vi "can test.vi"() -> ()   [LabVIEW 2015]
uses:
  <vilib>/myRIO/Instrument Drivers/Onboard IO/DIO/typedefs/DIO Reference.ctl
  <vilib>/myRIO/Common/Instrument Driver Framework/Utilities/typedefs/myRIO Generic Hardware Reference.ctl
  <vilib>/myRIO/Common/Instrument Driver Framework/Utilities/typedefs/Hardware Version Enum.ctl
  <vilib>/myRIO/Common/Instrument Driver Framework/Utilities/typedefs/myRIO v1.0 Reference.ctl
  <vilib>/myRIO/Common/Instrument Driver Framework/Utilities/typedefs/Generic FPGA Reference.ctl
  <vilib>/myRIO/Common/Instrument Driver Framework/myRIO v1.0/DIO/typedefs/DIO Channels List.ctl
  <vilib>/myRIO/Common/Instrument Driver Framework/myRIO v1.0/DIO/typedefs/DIO Channels Enum.ctl
  <vilib>/userdefined/High Color/nirio_resource_hc.ctl
  <vilib>/myRIO/Common/Instrument Driver Framework/myRIO v1.0/DIO/vis/myRIO v1.1 Open DIO.vi
  <vilib>/myRIO/Common/Instrument Driver Framework/Utilities/vis/Validate Channels.vi
  <vilib>/myRIO/Common/Instrument Driver Framework/myRIO v1.0/DIO/vis/myRIO v1.0 Reserve DIO.vi
  <vilib>/myRIO/Common/Instrument Driver Framework/myRIO v1.0/PWM/vis/myRIO v1.0 Close PWM.vi
  <vilib>/myRIO/Common/Instrument Driver Framework/myRIO v1.0/AO/vis/myRIO v1.0 Close AO.vi
  <vilib>/myRIO/Common/Instrument Driver Framework/myRIO v1.0/DIO/vis/myRIO v1.0 Close DIO.vi
  <vilib>/myRIO/Common/Instrument Driver Framework/myRIO v1.0/Resource Manager/vis/myRIO v1.0 Reserve Channel List.vi
  <vilib>/myRIO/Common/Instrument Driver Framework/myRIO v1.0/DIO/vis/myRIO v1.0 Build MUX Configuration DIO.vi
  <vilib>/myRIO/Common/Instrument Driver Framework/myRIO v1.0/PWM/vis/myRIO v1.0 Unreserve PWM.vi
  <vilib>/myRIO/Common/Instrument Driver Framework/myRIO v1.0/AO/vis/myRIO v1.0 Unreserve AO.vi
  <vilib>/myRIO/Common/Instrument Driver Framework/myRIO v1.0/DIO/vis/myRIO v1.0 Unreserve DIO.vi
  <vilib>/myRIO/Common/Instrument Driver Framework/myRIO v1.0/Resource Manager/vis/myRIO v1.0 Reserve Channel.vi
  <vilib>/myRIO/Common/Instrument Driver Framework/myRIO v1.0/Resource Manager/vis/myRIO v1.0 Unreserve Channel.vi
  <vilib>/myRIO/Common/Instrument Driver Framework/myRIO v1.0/Resource Manager/vis/myRIO v1.0 Create Configuration List.vi
  <vilib>/myRIO/Common/Instrument Driver Framework/myRIO v1.0/PWM/vis/myRIO v1.0 Build MUX Configuration PWM.vi
  <vilib>/myRIO/Common/Instrument Driver Framework/myRIO v1.0/Resource Manager/vis/myRIO v1.0 Unreserve Channel List.vi
  <vilib>/myRIO/Common/Instrument Driver Framework/myRIO v1.0/AO/vis/myRIO v1.0 Build MUX Configuration AO.vi
  <vilib>/myRIO/Common/Instrument Driver Framework/myRIO v1.0/Resource Manager/vis/myRIO v1.0 Build Mutex Name.vi
  rio_Global.vi
  <vilib>/Utility/VariantDataType/GetNumericInfo.vi
  <vilib>/Utility/error.llb/Error Cluster From Error Code.vi
  <vilib>/myRIO/Common/Instrument Driver Framework/myRIO v1.0/myRIO v1.1 Open.vi
  <vilib>/myRIO/Common/Instrument Driver Framework/Utilities/vis/IO Manager.vi
  <vilib>/myRIO/Common/Instrument Driver Framework/Utilities/vis/Configuration Manager.vi
  <vilib>/myRIO/Common/Instrument Driver Framework/myRIO v1.0/Resource Manager/vis/myRIO v1.0 Configure IO.vi
  <vilib>/myRIO/Common/Instrument Driver Framework/myRIO v1.0/myRIO v1.0 Close.vi
  <vilib>/myRIO/Common/Instrument Driver Framework/myRIO v1.0/DIO/vis/myRIO v1.0 Read DIO.vi
  <vilib>/myRIO/Common/Instrument Driver Framework/myRIO v1.0/PWM/vis/myRIO v1.0 Write PWM.vi
  <vilib>/myRIO/Common/Instrument Driver Framework/myRIO v1.0/AO/vis/myRIO v1.0 Write AO.vi
  <vilib>/myRIO/Common/Instrument Driver Framework/myRIO v1.0/DIO/vis/myRIO v1.0 Write DIO.vi
  <vilib>/myRIO/Common/Instrument Driver Framework/myRIO v1.0/PWM/vis/myRIO v1.0 Shutdown PWM.vi
  <vilib>/myRIO/Common/Instrument Driver Framework/myRIO v1.0/DIO/vis/myRIO v1.0 Shutdown DIO.vi
  <vilib>/Analysis/Matrix/Numeric/Conversions/Array To Matrix - RA2.vi
  <vilib>/Analysis/Matrix/Numeric/Multiply/Multiply - RM,RM.vi
  <vilib>/Analysis/Matrix/Numeric/Add/Add - RM,RM.vi
  <vilib>/Analysis/baseanly.llb/Real Inverse Matrix.vi
  <vilib>/Analysis/Matrix/Numeric/Subtract/Subtract - RM,RM.vi
  <vilib>/Analysis/Matrix/Numeric/Conversions/Array To Matrix - RA.vi
  <vilib>/Analysis/Matrix/Numeric/Multiply/Multiply - R,RM.vi
  <vilib>/Analysis/Matrix/Numeric/Conversions/Matrix To Array - RM.vi
  <vilib>/myRIO/Instrument Drivers/Onboard IO/DIO/vis/myRIO DIO Open.xnode
  <vilib>/myRIO/Instrument Drivers/Onboard IO/DIO/DIO.lvlib
  <vilib>/myRIO/Instrument Drivers/Onboard IO/PWM/PWM.lvlib
  <vilib>/myRIO/Instrument Drivers/Onboard IO/AO/AO.lvlib
  <vilib>/Analysis/Matrix/NI_Matrix.lvlib
  <vilib>/Analysis/NI_AALBase.lvlib
panel:
  in  "upper limit":dbl=1.0 format="%#_13g"
  out "XY Graph":cluster{"Y":dbl[], "Y":dbl[]}[](graph)=[{"Y"=[1.82421875, 1.8301353427767753, 1.835194070339203, 1.8394013252854347, 1.8427635002136231, 1.84528698772192, 1.8469781804084777, 1.8478434708714486, 1.8478892517089844, 1.8471219155192375, 1.84554785490036, 1.8431734624505043, 1.8400051307678222, 1.8360492524504661, 1.8313122200965881, 1.8258004263043404, 1.819520263671875, 1.8124781247973443, 1.8046804022789003, 1.796133488714695, 1.7868437767028809, 1.77681765884161, 1.7660615277290344, 1.7545817759633064, 1.742384796142578, 1.7294769808650017, 1.7158647227287291, 1.701554414331913, 1.686552448272705, 1.6708652171492577, 1.654499113559723, 1.637460530102253, 1.619755859375, 1.6013914939761162, 1.5823738265037537, 1.5627092495560646, 1.5424041557312012, 1.5214649376273155, 1.4998979878425598, 1.4777096989750862, 1.4549064636230469, 1.431494674384594, 1.4074807238578795, 1.3828710046410562, 1.3576719093322753, 1.3318898305296898, 1.3055311608314515, 1.2786022928357124, 1.251109619140625, 1.2230595323443412], "Y"=[0.0, 0.5, 1.0, 1.5, 2.0, 2.5, 3.0, 3.5, 4.0, 4.5, 5.0, 5.5, 6.0, 6.5, 7.0, 7.5, 8.0, 8.5, 9.0, 9.5, 10.0, 10.5, 11.0, 11.5, 12.0, 12.5, 13.0, 13.5, 14.0, 14.5, 15.0, 15.5, 16.0, 16.5, 17.0, 17.5, 18.0, 18.5, 19.0, 19.5, 20.0, 20.5, 21.0, 21.5, 22.0, 22.5, 23.0, 23.5, 24.0, 24.5]}, {"Y"=[-1.22265625, -1.2167396572232247, -1.211680929660797, -1.2074736747145653, -1.2041114997863769, -1.20158801227808, -1.1998968195915223, -1.1990315291285514, -1.1989857482910156, -1.1997530844807625, -1.20132714509964, -1.2037015375494957, -1.2068698692321778, -1.2108257475495339, -1.2155627799034119, -1.2210745736956596, -1.227354736328125, -1.2343968752026557, -1.2421945977210997, -1.250741511285305, -1.2600312232971191, -1.27005734115839, -1.2808134722709656, -1.2922932240366936, -1.304490203857422, -1.3173980191349983, -1.3310102772712709, -1.345320585668087, -1.360322551727295, -1.3760097828507423, -1.392375886440277, -1.409414469897747, -1.427119140625, -1.4454835060238838, -1.4645011734962463, -1.4841657504439354, -1.5044708442687988, -1.5254100623726845, -1.5469770121574402, -1.5691653010249138, -1.5919685363769531, -1.615380325615406, -1.6393942761421205, -1.6640039953589438, -1.6892030906677247, -1.7149851694703102, -1.7413438391685485, -1.7682727071642876, -1.795765380859375, -1.8238154676556588, -1.8524165749549866, -1.8815623101592065, -1.911246280670166, -1.9414620938897134, -1.972203357219696, -2.003463678061962, -2.0352366638183597, -2.0675159218907355, -2.1002950596809384, -2.1335676845908162, -2.167327404022217, -2.2015678253769875, -2.2362825560569766, -2.2714652034640315, -2.307109375, -2.3432086780667305, -2.3797567200660703, -2.4167471083998677, -2.4541734504699706, -2.4920293536782263, -2.530308425426483, -2.5690042731165885, -2.6081105041503907, -2.647620725929737, -2.687528545856476, -2.7278275713324547, -2.7685114097595216, -2.809573668539524, -2.8510079550743104, -2.892807876765728, -2.934967041015625, -2.977479055225849, -3.020337526798248, -3.0635360631346704, -3.107068271636963, -3.150927759706974, -3.1951081347465515, -3.2396030041575434, -3.284405975341797, -3.3295106557011604, -3.3749106526374817, -3.4205995735526087, -3.466571025848389, -3.51281861692667, -3.5593359541893004], "Y"=[0.0, 0.5, 1.0, 1.5, 2.0, 2.5, 3.0, 3.5, 4.0, 4.5, 5.0, 5.5, 6.0, 6.5, 7.0, 7.5, 8.0, 8.5, 9.0, 9.5, 10.0, 10.5, 11.0, 11.5, 12.0, 12.5, 13.0, 13.5, 14.0, 14.5, 15.0, 15.5, 16.0, 16.5, 17.0, 17.5, 18.0, 18.5, 19.0, 19.5, 20.0, 20.5, 21.0, 21.5, 22.0, 22.5, 23.0, 23.5, 24.0, 24.5, 25.0, 25.5, 26.0, 26.5, 27.0, 27.5, 28.0, 28.5, 29.0, 29.5, 30.0, 30.5, 31.0, 31.5, 32.0, 32.5, 33.0, 33.5, 34.0, 34.5, 35.0, 35.5, 36.0, 36.5, 37.0, 37.5, 38.0, 38.5, 39.0, 39.5, 40.0, 40.5, 41.0, 41.5, 42.0, 42.5, 43.0, 43.5, 44.0, 44.5, 45.0, 45.5, 46.0, 46.5, 47.0]}, {"Y"=[-0.94, 0.94, 0.94, -0.94, -0.94], "Y"=[-3.2, -3.2, 1.5, 1.5, -3.2]}, {"Y"=[1.984375, 1.978057861328125, 1.9718017578125, 1.965606689453125, 1.95947265625], "Y"=[0.0, 0.5, 1.0, 1.5, 2.0]}, {"Y"=[-5.28125, -5.267578125, -5.25390625, -5.240234375, -5.2265625], "Y"=[0.0, 0.5, 1.0, 1.5, 2.0]}]
  out "Heading":dbl
  out "H_GPS":dbl
  out "pos":dbl[](array[numeric])
  in  "GPS init":bool=TRUE
  out "pos_gps":dbl[](array[numeric]) format="%#_19f"
  out "dt":dbl
  out "Pos_time 10":i32
  out "ecef ref":dbl[](array[numeric])
  out "map":i32=2
  out "vgain":dbl=1.0
  out "vcount":u64=1
  out "hbias":dbl
  out "hcount":u64=1
  out "get heading":bool
  out "get position":bool
  out "heading error":dbl
  out "h_gps":dbl
  out "rt":dbl
  out "pos error":dbl
  out "POS init":bool
  out "Numeric":dbl
  out "cmd steer":dbl=25.77230806 format="%#_12g"
  in  "lane center":dbl=0.05 format="%#_13g"
  in  "Kf":dbl=0.18 format="%#_13g"
  out "Waveform Chart":dynamicdata(graph)
  out "mdps torque volt":dbl
  out "recomammed Speed [km/h]":dbl
  out "lane both":bool
  in  "gain(<1)":dbl=1.0 format="%#_13g"
  in  "rate limit":dbl=0.006 format="%#_13g"
  in  "deadzone":dbl
  in  "visco":dbl
  in  "Kp":dbl=1.2 format="%#_13g"
  out "VS_CAN":dbl
  out "car":refnum<k5>
  in  "forgetting":dbl format="%#_13g"
  out "mdps str_ang":dbl
  out "eye":refnum<k5>
  out "APV":dbl
  out "PWM GAS":dbl=1000.0 min=1000.0 max=2000.0 step=1.0
  out "Auto":bool
  in  "Manual Steering torque":dbl(slide) min=-0.3 max=0.3 step=0.01 scale=-0.3..0.3
  in  "Steering torque input":bool
  out "T init":i32
  out "T out":i32
  in  "manual speed":dbl
  in  "Velocity input":bool
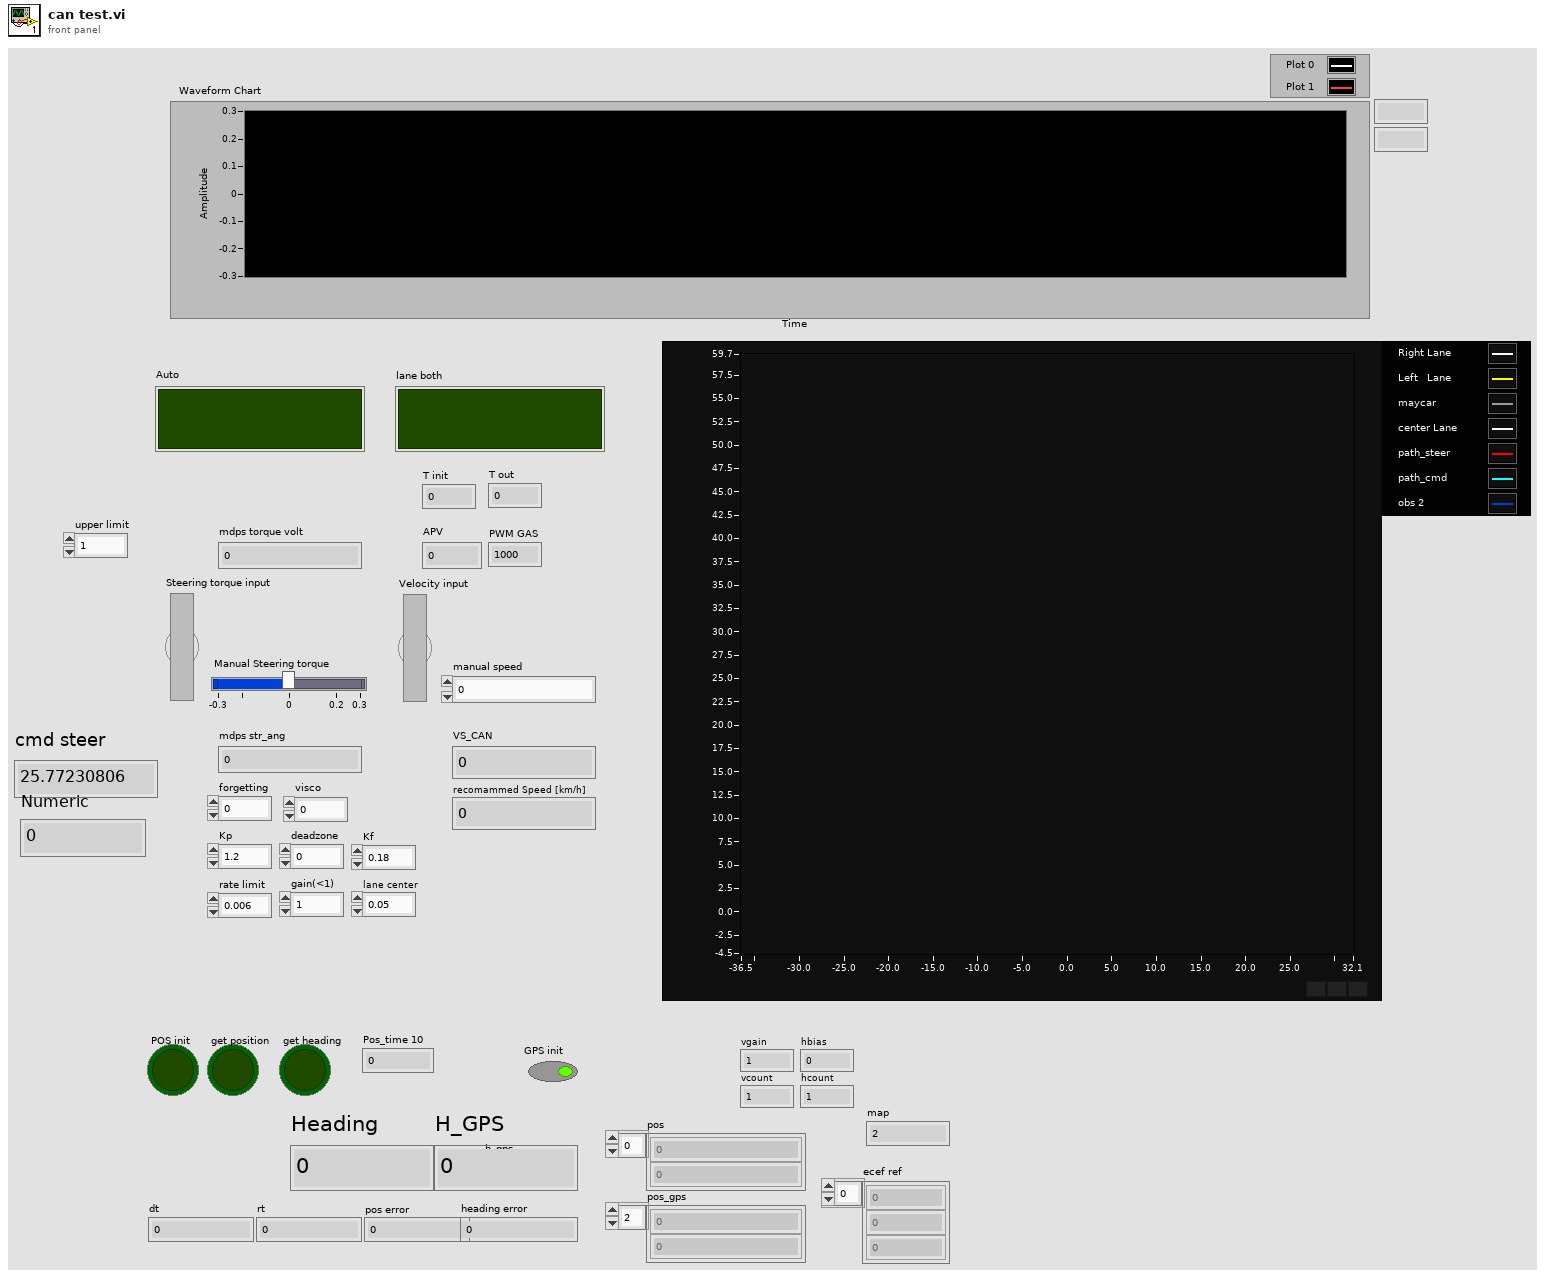
[diagram p1: front panel]
types:
  T1 = enum16{"Standard", "Buffered", "CRLF", "Immediate"}
  T2 = cluster{"identifier":u32, "timestamp":timestamp, "payload":u8[]}
  T3 = typedef "nirio_resource_hc.ctl" = tag
  T4 = typedef "Hardware Version Enum.ctl" = enum16{"Unknown", "myRIO-1900", "myRIO-1950", "roboRIO"}
  T5 = cluster{"connection ID":refnum<k16>, "net address":u32, "port":u16}
  T6 = cluster{"hash":i64, "sys time":i64, "mobileye time":u32, "ID":u32, "data":u8[]}
  T7 = cluster{"hash":i64, "sys time":i64, "car time":u32, "ID":u32, "data":u8[]}
  T8 = typedef "PWM.lvlib/PWM Reference.ctl" = cluster{"myRIO Reference":T9, "PWM Channels Enum":T12, "PWM Configuration":T13}
  T9 = typedef "myRIO Generic Hardware Reference.ctl" = cluster{"myRIO Model":T4, "myRIO Hardware Reference":T10}
  T10 = typedef "myRIO v1.0 Reference.ctl" = cluster{"Generic FPGA Reference":T11, "Allow multiple opens":bool}
  T11 = typedef "Generic FPGA Reference.ctl" = refnum<k20>
  T12 = typedef "PWM Channels Enum.ctl" = enum16{"Not Connected", "C/PWM0", "C/PWM1", "A/PWM0", "A/PWM1", "A/PWM2", "B/PWM0", "B/PWM1", "B/PWM2", "PWM/PWM0", "PWM/PWM1", "PWM/PWM2", "PWM/PWM3", "PWM/PWM4", "PWM/PWM5", "PWM/PWM6", "PWM/PWM7", "PWM/PWM8", "PWM/PWM9"}
  T13 = typedef "PWM.lvlib/PWM Configuration.ctl" = cluster{"Frequency":dbl, "Duty Cycle":dbl}
  T14 = typedef "DIO.lvlib/DIO Reference.ctl" = cluster{"myRIO Reference":T9, "DIO Channels List":T15}
  T15 = typedef "DIO Channels List.ctl" = T16[]
  T16 = typedef "DIO Channels Enum.ctl" = enum16{"Not Connected", "C/DIO0", "C/DIO1", "C/DIO2", "C/DIO3", "C/DIO4", "C/DIO5", "C/DIO6", "C/DIO7", "A/DIO0", "A/DIO1", "A/DIO2", "A/DIO3", "A/DIO4", "A/DIO5", "A/DIO6", "A/DIO7", "A/DIO8", "A/DIO9", "A/DIO10", "A/DIO11", "A/DIO12", "A/DIO13", "A/DIO14", "A/DIO15", "B/DIO0", "B/DIO1", "B/DIO2", "B/DIO3", "B/DIO4", "B/DIO5", "B/DIO6", "B/DIO7", "B/DIO8", "B/DIO9", "B/DIO10", "B/DIO11", "B/DIO12", "B/DIO13", "B/DIO14", "B/DIO15", "LED0", "LED1", "LED2", "LED3", "Button0", "DIO/DIO0", "DIO/DIO1", "DIO/DIO2", "DIO/DIO3", "DIO/DIO4", "DIO/DIO5", "DIO/DIO6", "DIO/DIO7", "DIO/DIO8", "DIO/DIO9", "SPI/CS0", "SPI/CS1", "SPI/CS2", "SPI/CS3", "LED RADIO (Green)", "LED RADIO (Red)", "LED COMM (Green)", "LED COMM (Red)", "LED MODE (Green)", "LED MODE (Red)"}
  T17 = typedef "AO.lvlib/AO Reference.ctl" = cluster{"myRIO Reference":T9, "AO Channel List":T18, "AO Scaling Constant List":T20}
  T18 = typedef "AO Channels List.ctl" = T19[]
  T19 = typedef "AO Channels Enum.ctl" = enum16{"Not Connected", "AudioOut/Left", "AudioOut/Right", "C/AO0", "C/AO1", "A/AO0", "A/AO1", "B/AO0", "B/AO1"}
  T20 = typedef "Analog Scaling Constants List.ctl" = T21[]
  T21 = typedef "Analog Scaling Constants.ctl" = cluster{"LSB Weight (Volts)":dbl, "Offset (Volts)":dbl, "Signed?":bool}
  T22 = cluster{"hash":i64, "sys time":i64, "ref_vel":dbl, "ref_steer":dbl}
  T23 = cluster{"hash":i64, "sys time":i64, "time":dbl, "x":dbl, "y":dbl, "h":dbl, "numSV":i32, "postype":i32, "lag":i32, "hordev":dbl, "lat":dbl, "lon":dbl, "hgt":dbl, "map_idx":i32}
  T24 = cluster{"output[0]":dbl, "output[1]":dbl, "output[2]":dbl, "output[3]":dbl, "output[4]":dbl, "output[5]":dbl, "output[6]":dbl, "output[7]":dbl, "output[8]":dbl, "output[9]":dbl, "output[10]":dbl, "output[11]":dbl, "output[12]":dbl, "output[13]":dbl, "output[14]":dbl}
  T25 = cluster{"hash":i64, "sys time":i64, "time":dbl, "speed":dbl, "heading":dbl, "lat":dbl, "lon":dbl}
  T26 = cluster{"output[0]":dbl, "output[1]":dbl, "output[2]":dbl, "output[3]":dbl, "output[4]":dbl, "output[5]":dbl, "output[6]":dbl}
  T27 = typedef "NI_Matrix.lvlib/RealMatrix.ctl" = dbl[][]
  T28 = cluster{"hash":i64, "sys time":i64, "dt":dbl, "x":dbl, "y":dbl, "speed":dbl, "heading":dbl, "yaw_rate":dbl}
  T29 = cluster{"Real 2D Array[0]":dbl, "Real 2D Array[1]":dbl, "Real 2D Array[2]":dbl, "Real 2D Array[3]":dbl, "Real 2D Array[4]":dbl}
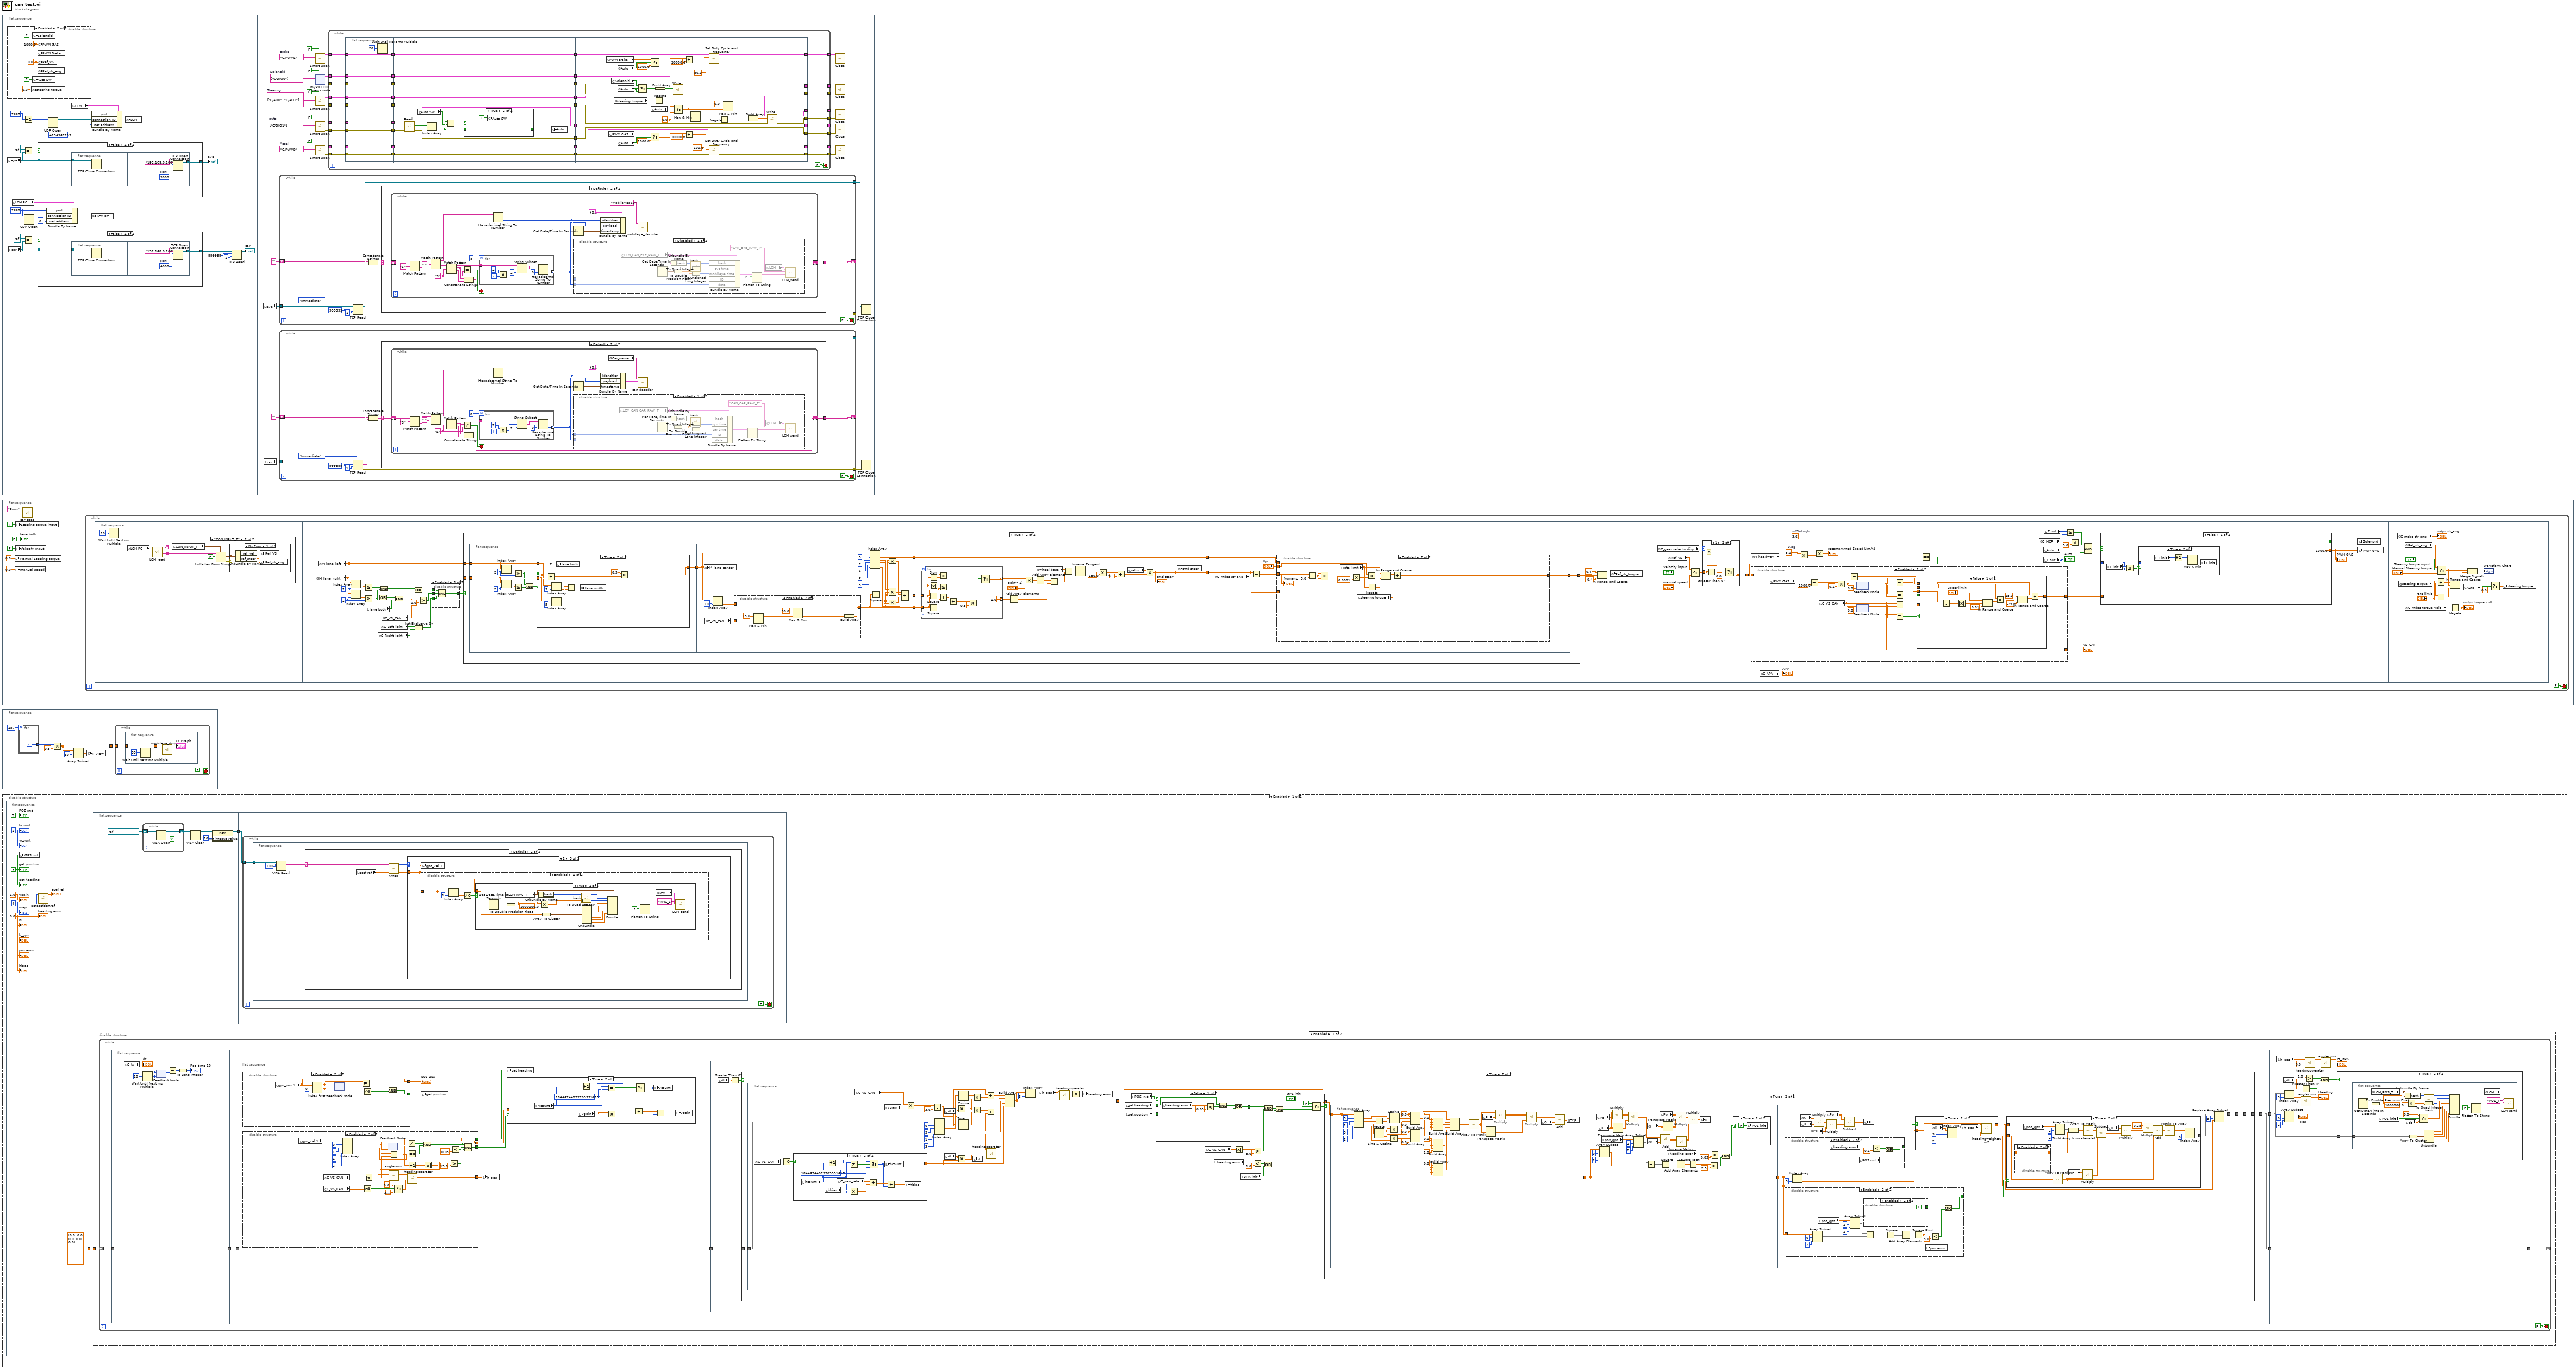
[diagram p0: block diagram]
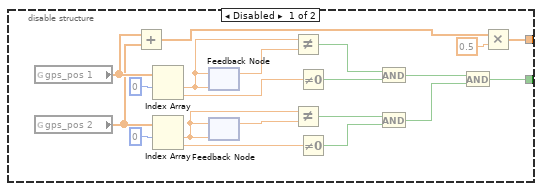
[diagram p2: hidden frame]
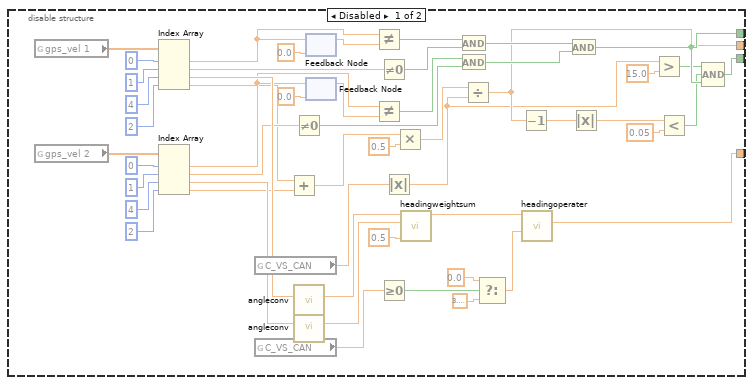
[diagram p3: hidden frame]
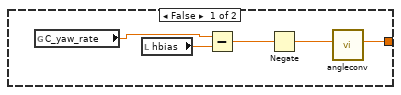
[diagram p6: hidden frame]
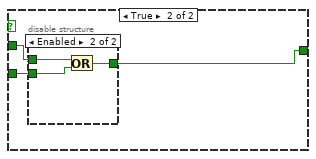
[diagram p7: hidden frame]
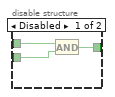
[diagram p8: hidden frame]
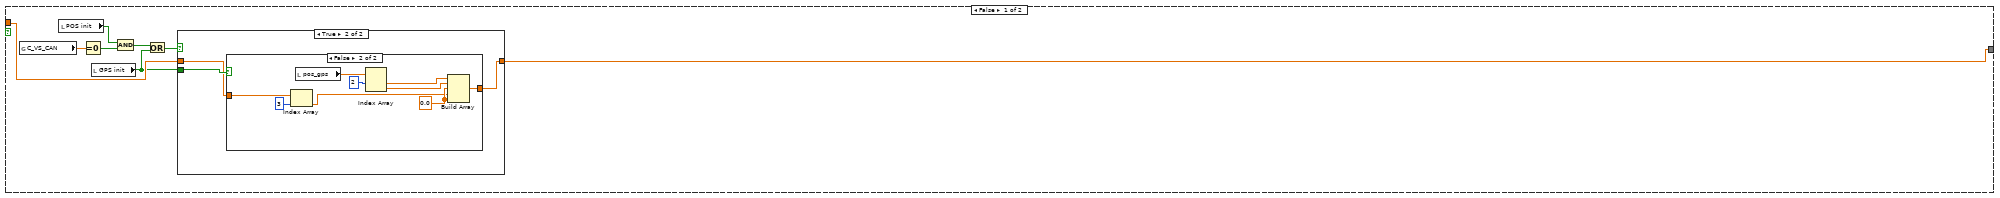
[diagram p9: hidden frame]
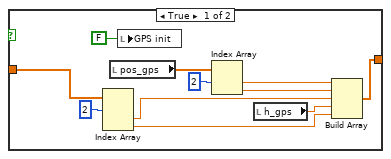
[diagram p11: hidden frame]
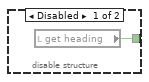
[diagram p13: hidden frame]
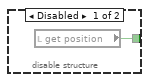
[diagram p14: hidden frame]
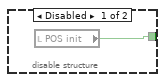
[diagram p15: hidden frame]
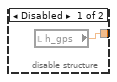
[diagram p17: hidden frame]
diagram:
  n1 = flat-sequence {
    frame #0 {
      w16 = u16 7668 ("port")
      w11 = u16 7667 ("port")
      n2 = disable-structure shown="Enabled" {
        frame Disabled {
        }
        frame Enabled {
          w24 = 0.0 ("Ref_str_ang")
          w25 = 1000.0 ("PWM GAS")
          n3 = global write "rio_Global.vi" "steering torque"(0.0 ("steering")) -> ()
          n4 = global write "rio_Global.vi" "Solenoid"(FALSE ("CAN A 1")) -> ()
          n5 = global write "rio_Global.vi" "Auto SW"(FALSE ("Auto SW")) -> ()
          n6 = global write "rio_Global.vi" "PWM GAS"(w25) -> ()
          n7 = global write "rio_Global.vi" "PWM Brake"(w25) -> ()
          n8 = global write "rio_Global.vi" "Ref_VS"(w24) -> ()
          n9 = global write "rio_Global.vi" "Ref_str_ang"(w24) -> ()
        }
      }
      n10 = local read "eye"() -> (w18:refnum<k5>)
      n11 = local read "car"() -> (w19:refnum<k5>)
      n12 = global read "rio_Global.vi" "LCM PC"() -> (w8:T5)
      n13 = Equal?(x=refnum<k5> refnum ("connection ID"), y=w18) -> (x = y?=w20:bool)
      n14 = Equal?(x=refnum<k5> refnum ("connection ID"), y=w19) -> (x = y?=w22:bool)
      n15 = Decrement(x=w11) -> (x-1=w10:u16)
      n16 = UDP Open(11:w16) -> (port=w14:refnum<k16>)  [unwired: 4 in, 2 out]
      n17 = case shown="False" w20 {
        tunnel: w18 -> [w30 _]
        tunnel: [w29 w35] -> w17
        frame False {
          n18 = flat-sequence {
            tunnel: w30 -> [w31]
            tunnel: [w32] -> w29
            frame #0 {
              n19 = TCP Close Connection(connection ID=w31) -> ()  [unwired: 2 in, 2 out]
            }
            frame #1 {
              w33 = u16 3000  # port
              n20 = TCP Open Connection(address="192.168.0.100", remote port or service name=w33) -> (connection ID=w32:refnum<k5>)  [unwired: 3 in, 1 out]
            }
          }
        }
        frame True {
          w36 = u16 3000  # port
          n21 = TCP Open Connection(address="192.168.0.100", remote port or service name=w36) -> (connection ID=w35:refnum<k5>)  [unwired: 3 in, 1 out]
        }
      }
      "eye" <- w17
      n22 = case shown="False" w22 {
        tunnel: w19 -> [w39 _]
        tunnel: [w38 w44] -> w3
        frame False {
          n23 = flat-sequence {
            tunnel: w39 -> [w40]
            tunnel: [w41] -> w38
            frame #0 {
              n24 = TCP Close Connection(connection ID=w40) -> ()  [unwired: 2 in, 2 out]
            }
            frame #1 {
              w42 = u16 4000  # port
              n25 = TCP Open Connection(address="192.168.0.200", remote port or service name=w42) -> (connection ID=w41:refnum<k5>)  [unwired: 3 in, 1 out]
            }
          }
        }
        frame True {
          w45 = u16 4000  # port
          n26 = TCP Open Connection(address="192.168.0.200", remote port or service name=w45) -> (connection ID=w44:refnum<k5>)  [unwired: 3 in, 1 out]
        }
      }
      n27 = Bundle By Name(cluster=w8, "port"=w16, "connection ID"=w14, "net address"=u32 0) -> (w9:T5)
      n28 = UDP Open(11:w10) -> (port=w13:refnum<k16>)  [unwired: 4 in, 2 out]
      n29 = global read "rio_Global.vi" "LCM"() -> (w7:T5)
      n30 = Bundle By Name(cluster=w7, "port"=w11, "connection ID"=w13, "net address"=u32 4294967295) -> (w6:T5)
      n31 = global write "rio_Global.vi" "LCM PC"(w9) -> ()
      n32 = global write "rio_Global.vi" "LCM"(w6) -> ()
      n33 = TCP Read(connection ID=w3, bytes to read=999999, 9:1 ("timeout ms (25000)")) -> (connection ID out=→"car":refnum<k5>)  [unwired: 2 in, 2 out]
    }
    frame #1 {
      w50 = tag "C/PWM1"  # Brake
      w64 = tag[] ["C/AO0", "C/AO1"]  # Steering
      w71 = tag[] ["C/DIO1"]  # auto
      w76 = tag "C/PWM0"  # Accel
      w81 = tag[] ["C/DIO0"]  # Solenoid
      n34 = local read "eye"() -> (w55:refnum<k5>)
      n35 = local read "car"() -> (w51:refnum<k5>)
      n36 = while {
        tunnel: w55 -> [w140]
        tunnel: [w142] -> w58
        tunnel: [w141] -> w57
        shift-right: [w136] -> _
        shift-left: "" -> [w139]
        stop <- FALSE stop-if-true
        n37 = TCP Read(connection ID=w140, bytes to read=999999, 7:T1."Immediate" ("mode (standard)"), 9:1 ("timeout ms (25000)")) -> (connection ID out=w142:refnum<k5>, data out=w138:string, error out=w141:errorcluster)  [unwired: 1 in]
        n38 = Concatenate Strings(w139, w138) -> (w137:string)
        n39 = case shown="Default" w137 {
          selector: w137 -> [_ w148]
          tunnel: [_ w147] -> w136
          frame "" {
          }
          frame Default {
            n40 = while {
              shift-right: [w155] -> w147
              shift-left: w148 -> [w167]
              stop <- w152 stop-if-true
              w153 = "S" ("regular expression")
              n41 = Match Pattern(string=w167, regular expression="S") -> (after substring=w165:string)  [unwired: 1 in, 3 out]
              n42 = Match Pattern(string=w165, regular expression=" ") -> (before substring=w163:string, after substring=w160:string)  [unwired: 1 in, 2 out]
              n43 = Match Pattern(string=w160, regular expression=w153) -> (before substring=w159:string, match substring=w154:string, after substring=w156:string)  [unwired: 1 in, 1 out]
              n44 = Not Equal?(x=w154, y=w153) -> (x != y?=w152:bool)
              n45 = Concatenate Strings(w154, w156) -> (w155:string)
              n46 = for {
                N: 8 -> [_]
                tunnel: w159 -> [w189]
                tunnel: [w185] -> w149 mode=indexing
                i -> [w184]
                n47 = Multiply(x=2, y=w184) -> (x*y=w187:i32)
                n48 = String Subset(string=w189, offset (0)=w187, length (rest)=2 ("length (rest)")) -> (substring=w182:string)
                n49 = Hexadecimal String To Number(string=w182, default (0uL)=u8 0) -> (number=w185:u8)  [unwired: 1 in, 1 out]
              }
              n50 = Hexadecimal String To Number(string=w163) -> (number=w150:u32)  [unwired: 2 in, 1 out]
              n51 = Get Date/Time In Seconds() -> (seconds since 1Jan1904=w158:timestamp)
              n52 = disable-structure shown="Disabled" {
                disable-tunnel: w150 -> [w169 _]
                disable-tunnel: w149 -> [w168 _]
                frame Disabled {
                  n53 = global read "rio_Global.vi" "LCM_CAN_EYE_RAW_T"() -> (w176:T6)
                  n54 = Get Date/Time In Seconds() -> (seconds since 1Jan1904=w173:timestamp)
                  n55 = Unbundle By Name(w176) -> ("hash"=w175:i64)
                  n56 = To Double Precision Float(number=w173) -> (double precision float=w171:dbl)
                  n57 = call "hash.vi"("input"=w175) -> ("output"=w177:i64)  [unwired: 10 in]
                  n58 = To Quad Integer(1:w171) -> (0:w172:i64)
                  n59 = To Unsigned Long Integer(number=w171) -> (unsigned 32bit integer=w170:u32)
                  n60 = Bundle By Name(cluster=w176, "hash"=w177, "sys time"=w172, "mobileye time"=w170, "ID"=w169, "data"=w168) -> (w179:T6)
                  n61 = Flatten To String(anything=w179, prepend array or string size? (T)=FALSE) -> (data string=w181:string)  [unwired: 2 in, 2 out]
                  n62 = global read "rio_Global.vi" "LCM"() -> (w180:T5)
                  n63 = call "LCM_send.vi"("DATA"=w181, "ID"="CAN_EYE_RAW_T", "LCM"=w180) -> ()  [unwired: 6 in, 3 out]
                }
                frame Enabled {
                }
              }
              n64 = Bundle By Name(cluster=T2 {"identifier"=0, "timestamp"=timestamp(0 s since 1904-01-01), "payload"=[]} ("can cluster"), "identifier"=w150, "payload"=w149, "timestamp"=w158) -> (w157:T2)
              n65 = call "mobileye_decoder.vi"("can cluster"=w157, "name"="Mobileye560") -> ()  [unwired: 10 in]
            }
          }
        }
      }
      n66 = while {
        tunnel: w51 -> [w87]
        tunnel: [w89] -> w52
        tunnel: [w88] -> w53
        shift-right: [w83] -> _
        shift-left: "" -> [w86]
        stop <- FALSE stop-if-true
        n67 = TCP Read(connection ID=w87, bytes to read=999999, 7:T1."Immediate" ("mode (standard)"), 9:1 ("timeout ms (25000)")) -> (connection ID out=w89:refnum<k5>, data out=w85:string, error out=w88:errorcluster)  [unwired: 1 in]
        n68 = Concatenate Strings(w86, w85) -> (w84:string)
        n69 = case shown="Default" w84 {
          selector: w84 -> [_ w95]
          tunnel: [_ w94] -> w83
          frame "" {
          }
          frame Default {
            n70 = while {
              shift-right: [w104] -> w94
              shift-left: w95 -> [w114]
              stop <- w100 stop-if-true
              w101 = "S" ("regular expression")
              n71 = Match Pattern(string=w114, regular expression="S") -> (after substring=w112:string)  [unwired: 1 in, 3 out]
              n72 = Match Pattern(string=w112, regular expression=" ") -> (before substring=w110:string, after substring=w108:string)  [unwired: 1 in, 2 out]
              n73 = Match Pattern(string=w108, regular expression=w101) -> (before substring=w107:string, match substring=w102:string, after substring=w105:string)  [unwired: 1 in, 1 out]
              n74 = Not Equal?(x=w102, y=w101) -> (x != y?=w100:bool)
              n75 = Concatenate Strings(w102, w105) -> (w104:string)
              n76 = for {
                N: 8 -> [_]
                tunnel: w107 -> [w135]
                tunnel: [w131] -> w97 mode=indexing
                i -> [w130]
                n77 = Multiply(x=2, y=w130) -> (x*y=w133:i32)
                n78 = String Subset(string=w135, offset (0)=w133, length (rest)=2 ("length (rest)")) -> (substring=w128:string)
                n79 = Hexadecimal String To Number(string=w128, default (0uL)=u8 0) -> (number=w131:u8)  [unwired: 1 in, 1 out]
              }
              n80 = Hexadecimal String To Number(string=w110) -> (number=w98:u32)  [unwired: 2 in, 1 out]
              n81 = Get Date/Time In Seconds() -> (seconds since 1Jan1904=w106:timestamp)
              n82 = disable-structure shown="Disabled" {
                disable-tunnel: w98 -> [w120 _]
                disable-tunnel: w97 -> [w119 _]
                frame Disabled {
                  n83 = global read "rio_Global.vi" "LCM_CAN_CAR_RAW_T"() -> (w125:T7)
                  n84 = Get Date/Time In Seconds() -> (seconds since 1Jan1904=w127:timestamp)
                  n85 = Unbundle By Name(w125) -> ("hash"=w126:i64)
                  n86 = To Double Precision Float(number=w127) -> (double precision float=w118:dbl)
                  n87 = call "hash.vi"("input"=w126) -> ("output"=w124:i64)  [unwired: 10 in]
                  n88 = To Quad Integer(1:w118) -> (0:w122:i64)
                  n89 = To Unsigned Long Integer(number=w118) -> (unsigned 32bit integer=w121:u32)
                  n90 = Bundle By Name(cluster=w125, "hash"=w124, "sys time"=w122, "car time"=w121, "ID"=w120, "data"=w119) -> (w123:T7)
                  n91 = Flatten To String(anything=w123) -> (data string=w115:string)  [unwired: 3 in, 2 out]
                  n92 = global read "rio_Global.vi" "LCM"() -> (w116:T5)
                  n93 = call "LCM_send.vi"("DATA"=w115, "ID"="CAN_CAR_RAW_T", "LCM"=w116) -> ()  [unwired: 6 in, 3 out]
                }
                frame Enabled {
                }
              }
              n94 = Bundle By Name(cluster=T2 {"identifier"=0, "timestamp"=timestamp(0 s since 1904-01-01), "payload"=[]} ("can cluster"), "identifier"=w98, "payload"=w97, "timestamp"=w106) -> (w103:T2)
              n95 = global read "rio_Global.vi" "Car_name"() -> (w96:string)
              n96 = call "can decoder.vi"("can cluster"=w103, "name"=w96) -> ()  [unwired: 10 in]
            }
          }
        }
      }
      n97 = call <vilib>:"Smart Open.vi"("Allow multiple opens?"=FALSE, "Channel Name"=w50) -> ("PWM Ref Out"=w48:T8)  [unwired: 8 in, 1 out]
      n98 = xnode "myRIO DIO Open.xnode"("Allow multiple opens?"=FALSE, "Channel Names"=w81) -> ("error out"=w79:errorcluster, "DIO Ref Out"=w80:T14)  [unwired: 1 in]
      n99 = call <vilib>:"Smart Open.vi"("Allow multiple opens?"=TRUE, "Channel Names"=w64) -> ("error out"=w62:errorcluster, "AO Ref Out"=w63:T17)  [unwired: 8 in]
      n100 = call <vilib>:"Smart Open.vi"("Allow multiple opens?"=FALSE, "Channel Names"=w71) -> ("error out"=w69:errorcluster, "DIO Ref Out"=w70:T14)  [unwired: 8 in]
      n101 = call <vilib>:"Smart Open.vi"("Allow multiple opens?"=FALSE, "Channel Name"=w76) -> ("error out"=w74:errorcluster, "PWM Ref Out"=w75:T8)  [unwired: 8 in]
      n102 = while {
        tunnel: w80 -> [w241]
        tunnel: [w242] -> w78
        tunnel: w79 -> [w240]
        tunnel: [w236] -> w77
        tunnel: w70 -> [w234]
        tunnel: [w232] -> w68
        tunnel: w69 -> [w233]
        tunnel: [w231] -> w67
        tunnel: w63 -> [w230]
        tunnel: [w228] -> w61
        tunnel: w62 -> [w229]
        tunnel: [w227] -> w60
        tunnel: w75 -> [w238]
        tunnel: [w239] -> w73
        tunnel: w74 -> [w237]
        tunnel: [w235] -> w72
        tunnel: w48 -> [w207]
        tunnel: [w206] -> w47
        stop <- FALSE ("Auto") stop-if-true
        n103 = flat-sequence {
          tunnel: w229 -> [w245]
          tunnel: w230 -> [w246]
          tunnel: w233 -> [w247]
          tunnel: w234 -> [w248]
          tunnel: w237 -> [w249]
          tunnel: w238 -> [w250]
          tunnel: w240 -> [w251]
          tunnel: w241 -> [w252]
          tunnel: [w252] -> w226
          tunnel: [w251] -> w224
          tunnel: [w250] -> w222
          tunnel: [w249] -> w220
          tunnel: [w248] -> w218
          tunnel: [w247] -> w216
          tunnel: [w246] -> w214
          tunnel: [w245] -> w212
          tunnel: [w243] -> w208
          tunnel: w207 -> [w243]
          tunnel: w226 -> [w268]
          tunnel: [w268] -> w225
          tunnel: w224 -> [w267]
          tunnel: [w267] -> w223
          tunnel: w222 -> [w266]
          tunnel: [w266] -> w221
          tunnel: w220 -> [w265]
          tunnel: [w265] -> w219
          tunnel: w218 -> [w261]
          tunnel: [w259] -> w217
          tunnel: w216 -> [w260]
          tunnel: [w258] -> w215
          tunnel: w214 -> [w264]
          tunnel: [w264] -> w213
          tunnel: w212 -> [w263]
          tunnel: [w263] -> w211
          tunnel: [w253] -> w209
          tunnel: w208 -> [w253]
          tunnel: [w314] -> w242
          tunnel: [w311] -> w239
          tunnel: [w308] -> w236
          tunnel: [w307] -> w235
          tunnel: [w293] -> w232
          tunnel: [w292] -> w231
          tunnel: [w303] -> w228
          tunnel: [w302] -> w227
          tunnel: w225 -> [w313]
          tunnel: w223 -> [w312]
          tunnel: w221 -> [w310]
          tunnel: w219 -> [w309]
          tunnel: w217 -> [w293]
          tunnel: w215 -> [w292]
          tunnel: w213 -> [w305]
          tunnel: w211 -> [w304]
          tunnel: w209 -> [w278]
          tunnel: [w277] -> w206
          frame #0 {
            n104 = Wait Until Next ms Multiple(millisecond multiple=u32 20) -> ()  [unwired: 1 out]
          }
          frame #1 {
            n105 = call <vilib>:"Read.vi"("error in (no error)"=w260, "DIO Ref In"=w261) -> ("error out"=w258:errorcluster, "Values"=w262:bool[], "DIO Ref Out"=w259:T14)  [unwired: 7 in]
            n106 = global read "rio_Global.vi" "Auto SW"() -> (w255:bool)
            n107 = Index Array(array=w262) -> (element=w256:bool)  [unwired: 1 in]
            n108 = Equal?(x=w256, y=w255) -> (x = y?=w257:bool)
            n109 = case shown="True" w257 {
              tunnel: w256 -> [_ w270]
              tunnel: [_ w270] -> w254
              frame False {
              }
              frame True {
                n110 = global write "rio_Global.vi" "Auto SW"(TRUE ("Auto SW")) -> ()
              }
            }
            n111 = global write "rio_Global.vi" "Auto"(w254) -> ()
          }
          frame #2 {
            w290 = 0.0 ("y")
            n112 = global read "rio_Global.vi" "PWM Brake"() -> (w274:dbl)
            n113 = global read "rio_Global.vi" "PWM GAS"() -> (w280:dbl)
            n114 = global read "rio_Global.vi" "Solenoid"() -> (w282:bool)
            n115 = global read "rio_Global.vi" "steering torque"() -> (w281:dbl)
            n116 = global read "rio_Global.vi" "Auto"() -> (w272:bool)
            n117 = global read "rio_Global.vi" "Auto"() -> (w283:bool)
            n118 = global read "rio_Global.vi" "Auto"() -> (w284:bool)
            n119 = Select(t=w282, s=w283, f=w283) -> (s? t:f=w286:bool)
            n120 = Select(t=w274, s=w272, f=1000.0) -> (s? t:f=w273:dbl)
            n121 = Select(t=w280, s=w284, f=1000.0) -> (s? t:f=w289:dbl)
            n122 = global read "rio_Global.vi" "Auto"() -> (w285:bool)
            n123 = Negate(x=w281) -> (-x=w287:dbl)
            n124 = Build Array(w286) -> (w297:bool[])
            n125 = call <vilib>:"Write.vi"("error in (no error)"=w312, "Values"=w297, "DIO Ref In"=w313) -> ("error out"=w308:errorcluster, "DIO Ref Out"=w314:T14)  [unwired: 6 in]
            n126 = Select(t=w287, s=w285, f=w290) -> (s? t:f=w291:dbl)
            n127 = Divide(x=w273, y=20000.0) -> (x/y=w276:dbl)
            n128 = Divide(x=w289, y=10000.0) -> (x/y=w294:dbl)
            n129 = Max & Min(x=w291, y=w290) -> (min(x,y)=w299:dbl)  [unwired: 1 out]
            n130 = call <vilib>:"Set Duty Cycle and Frequency.vi"("Frequency [Hz]"=50.0, "Duty Cycle"=w276, "PWM Ref In"=w278) -> ("PWM Ref Out"=w277:T8)  [unwired: 6 in, 1 out]
            n131 = call <vilib>:"Set Duty Cycle and Frequency.vi"("error in (no error)"=w309, "Frequency [Hz]"=100.0, "Duty Cycle"=w294, "PWM Ref In"=w310) -> ("error out"=w307:errorcluster, "PWM Ref Out"=w311:T8)  [unwired: 5 in]
            n132 = Negate(x=w299) -> (-x=w298:dbl)
            n133 = Max & Min(x=0.0, y=w291) -> (max(x,y)=w300:dbl)  [unwired: 1 out]
            n134 = Build Array(w300, w298) -> (w306:dbl[])
            n135 = call <vilib>:"Write.vi"("error in (no error)"=w304, "Values"=w306, "AO Ref In"=w305) -> ("error out"=w302:errorcluster, "AO Ref Out"=w303:T17)  [unwired: 6 in]
          }
        }
      }
      n136 = call <vilib>:"Close.vi"("PWM Ref In"=w47) -> ()  [unwired: 10 in, 1 out]
      n137 = call <vilib>:"Close.vi"("error in (no error)"=w77, "DIO Ref In"=w78) -> ()  [unwired: 9 in, 1 out]
      n138 = call <vilib>:"Close.vi"("error in (no error)"=w60, "AO Ref In"=w61) -> ()  [unwired: 9 in, 1 out]
      n139 = call <vilib>:"Close.vi"("error in (no error)"=w67, "DIO Ref In"=w68) -> ()  [unwired: 9 in, 1 out]
      n140 = call <vilib>:"Close.vi"("error in (no error)"=w72, "PWM Ref In"=w73) -> ()  [unwired: 9 in, 1 out]
      n141 = TCP Close Connection(connection ID=w58, error in (no error)=w57) -> ()  [unwired: 1 in, 2 out]
      n142 = TCP Close Connection(connection ID=w52, error in (no error)=w53) -> ()  [unwired: 1 in, 2 out]
    }
  }
  n143 = flat-sequence {
    frame #0 {
      n144 = local write "Manual Steering torque"(0.0 ("con_vs")) -> ()
      n145 = local write "manual speed"(0.0 ("manual speed")) -> ()
      n146 = local write "Steering torque input"(TRUE ("Steering torque input")) -> ()
      n147 = local write "Velocity input"(FALSE ("Velocity input")) -> ()
      n148 = call "car_spec.vi"("Car_name"="Prius") -> ()  [unwired: 5 in, 6 out]
      "lane both" <- FALSE ("lane both")
    }
    frame #1 {
      n149 = while {
        stop <- FALSE stop-if-true
        n150 = flat-sequence {
          tunnel: [w564] -> w321
          tunnel: w321 -> [w576]
          frame #0 {
            n151 = Wait Until Next ms Multiple(millisecond multiple=u32 10) -> ()  [unwired: 1 out]
          }
          frame #1 {
            n152 = global read "rio_Global.vi" "LCM PC"() -> (w326:T5)
            n153 = call "LCM_read.vi"("LCM"=w326) -> ("data"=w324:string, "ID"=w325:string)  [unwired: 7 in, 2 out]
            n154 = case shown="\"CON_INPUT_T\"" w325 {
              tunnel: w324 -> [_ w327]
              frame "False", Default {
              }
              frame "CON_INPUT_T" {
                n155 = global read "rio_Global.vi" "CON_INPUT_T"() -> (w329:T22)
                n156 = Unflatten From String(type=w329, binary string=w327, data includes array or string size? (T)=FALSE) -> (value=w328:T22, error out=w330:errorcluster)  [unwired: 2 in, 1 out]
                n157 = case shown="No Error" w330 {
                  tunnel: w328 -> [w334 _]
                  frame No Error {
                    n158 = Unbundle By Name(w334) -> ("ref_vel"=w333:dbl, "ref_steer"=w332:dbl)
                    n159 = global write "rio_Global.vi" "Ref_VS"(w333) -> ()
                    n160 = global write "rio_Global.vi" "Ref_str_ang"(w332) -> ()
                  }
                  frame Error {
                  }
                }
              }
            }
          }
          frame #2 {
            w355 = 2 ("index")
            w357 = 2 ("index")
            n161 = global read "rio_Global.vi" "M_lane_right"() -> (w340:dbl[])
            n162 = global read "rio_Global.vi" "M_lane_left"() -> (w339:dbl[])
            n163 = Index Array(array=w339, index=w357) -> (element=w358:dbl)
            n164 = Index Array(array=w340, index=w355) -> (element=w356:dbl)
            n165 = Greater Or Equal?(x=w358, y=w357) -> (x >= y?=w346:bool)
            n166 = Greater Or Equal?(x=w356, y=w355) -> (x >= y?=w347:bool)
            n167 = local read "lane both"() -> (w344:bool)
            n168 = global read "rio_Global.vi" "C_Right light"() -> (w336:bool)
            n169 = Or(x=w346, y=w347) -> (x .or. y?=w345:bool)
            n170 = And(x=w346, y=w347) -> (x .and. y?=w343:bool)
            n171 = global read "rio_Global.vi" "C_Left light"() -> (w337:bool)
            n172 = global read "rio_Global.vi" "C_VS_CAN"() -> (w338:dbl)
            n173 = And(x=w345, y=w344) -> (x .and. y?=w342:bool)
            n174 = Or(x=w343, y=w342) -> (x .or. y?=w341:bool)
            n175 = Not Exclusive Or(1:w336, 2:w337) -> (0:w353:bool)
            n176 = Greater?(x=w338, y=0.0) -> (0:w349:bool)
            n177 = disable-structure shown="Enabled" {
              disable-tunnel: [w362 TRUE] -> w354
              disable-tunnel: w353 -> [w361 _]
              disable-tunnel: w349 -> [w360 _]
              disable-tunnel: w341 -> [w359 _]
              frame Enabled {
                n178 = Compound Arithmetic op=AND(w359, w360, w361) -> (w362:bool)
              }
              frame Disabled {
              }
            }
            n179 = case shown="True" w354 {
              tunnel: [w367 w374] -> w350
              tunnel: w339 -> [_ w372]
              tunnel: w340 -> [_ w371]
              frame False {
                n180 = local write "lane both"(FALSE ("lane both")) -> ()
                n181 = global write "rio_Global.vi" "M_lane_center"(dbl[] [] ("M_lane_center")) -> ()
                n182 = global read "rio_Global.vi" "steering torque"() -> (w364:dbl)
                n183 = Multiply(x="forgetting", y=w364) -> (x*y=w367:dbl)
              }
              frame True {
                n184 = flat-sequence {
                  tunnel: [w381] -> w373
                  tunnel: w372 -> [w380]
                  tunnel: w371 -> [w379]
                  tunnel: [w429] -> w377
                  tunnel: [w428] -> w376
                  tunnel: w373 -> [w422]
                  tunnel: [w423] -> w369
                  tunnel: w377 -> [w483]
                  tunnel: w376 -> [w482]
                  tunnel: [w470] -> w375
                  tunnel: [w473] -> w370
                  tunnel: w369 -> [w473]
                  tunnel: w375 -> [w506]
                  tunnel: [w507] -> w374
                  tunnel: w370 -> [w504]
                  frame #0 {
                    w387 = 2 ("index")
                    w385 = 2 ("index")
                    n185 = Index Array(array=w380, index=w385) -> (element=w384:dbl)
                    n186 = Index Array(array=w379, index=w387) -> (element=w386:dbl)
                    n187 = Greater Or Equal?(x=w384, y=w385) -> (x >= y?=w378:bool)
                    n188 = Greater Or Equal?(x=w386, y=w387) -> (x >= y?=w383:bool)
                    n189 = And(x=w378, y=w383) -> (x .and. y?=w382:bool)
                    n190 = case shown="True" w382 {
                      tunnel: w380 -> [w409 w413]
                      tunnel: w379 -> [w404 w417]
                      tunnel: [w401 w418] -> w381
                      tunnel: w378 -> [w403 _]
                      frame False {
                        w396 = 0.2 ("y")
                        w399 = 5 ("index")
                        w408 = 5 ("index")
                        n191 = global read "rio_Global.vi" "overall width"() -> (w388:dbl)
                        n192 = Index Array(array=w409, index=w408) -> (element=w406:dbl)
                        n193 = Index Array(array=w404, index=w399) -> (element=w398:dbl)
                        n194 = global read "rio_Global.vi" "lane width"() -> (w389:dbl)
                        n195 = Multiply(x=w388, y=w396) -> (x*y=w394:dbl)
                        n196 = Add(x=w394, y=w396) -> (x+y=w390:dbl)
                        n197 = Add(x=1.0 ("y"), y=w394) -> (x+y=w391:dbl)
                        n198 = Multiply(x=w389, y=0.5) -> (x*y=w393:dbl)
                        n199 = In Range and Coerce(upper limit=w391, x=w393, lower limit=w390) -> (coerced(x)=w392:dbl)  [unwired: 1 out]
                        n200 = Add(x=w406, y=w392) -> (x+y=w405:dbl)
                        n201 = Subtract(x=w398, y=w392) -> (x-y=w397:dbl)
                        n202 = Replace Array Subset(array=w409, new element=w405, index=w408) -> (w402:dbl[])
                        n203 = Replace Array Subset(array=w404, new element=w397, index=w399) -> (w400:dbl[])
                        n204 = Select(t=w402, s=w403, f=w400) -> (s? t:f=w401:dbl[])
                      }
                      frame True {
                        n205 = Add(x=w413, y=w417) -> (x+y=w420:dbl[])
                        n206 = Index Array(array=w413, index=5) -> (element=w411:dbl)
                        n207 = Index Array(array=w417, index=5) -> (element=w415:dbl)
                        n208 = local write "lane both"(TRUE ("lane both")) -> ()
                        n209 = Subtract(x=w415, y=w411) -> (x-y=w410:dbl)
                        n210 = global write "rio_Global.vi" "lane width"(w410) -> ()
                        n211 = Multiply(x=0.5, y=w420) -> (x*y=w418:dbl[])
                      }
                    }
                  }
                  frame #1 {
                    n212 = global write "rio_Global.vi" "M_lane_center"(w422) -> ()
                    n213 = global read "rio_Global.vi" "C_VS_CAN"() -> (w421:dbl)
                    n214 = Index Array(array=w422, index=10) -> (element=w425:dbl)
                    n215 = disable-structure shown="Enabled" {
                      disable-tunnel: w421 -> [w462 w463]
                      disable-tunnel: [w453 w467] -> w428
                      disable-tunnel: w425 -> [w447 _]
                      frame Disabled {
                        n216 = Subtract(x=w447, y=15.0) -> (x-y=w445:dbl)
                        n217 = Subtract(x=w462, y=15.0) -> (x-y=w456:dbl)
                        n218 = Max & Min(x=w445, y=0.0) -> (max(x,y)=w444:dbl)  [unwired: 1 out]
                        n219 = Max & Min(x=w456, y=0.0) -> (max(x,y)=w455:dbl)  [unwired: 1 out]
                        n220 = Multiply(x=w444, y=2.0) -> (x*y=w452:dbl)
                        n221 = Multiply(x=w455, y=2.0) -> (x*y=w459:dbl)
                        n222 = Round Toward -Infinity(1:w452) -> (0:w443:dbl)
                        n223 = Round Toward -Infinity(1:w459) -> (0:w458:dbl)
                        n224 = Increment(x=w443) -> (x+1=w442:dbl)
                        n225 = Increment(x=w458) -> (x+1=w450:dbl)
                        n226 = global read "rio_Global.vi" "x_view"() -> (w441:dbl[])
                        n227 = Max & Min(x=w442, y=w450) -> (min(x,y)=w449:dbl)  [unwired: 1 out]
                        n228 = Array Subset(array=w441, index=0, length=w449) -> (w453:dbl[])
                      }
                      frame Enabled {
                        n229 = Max & Min(x=15.0, y=w463) -> (max(x,y)=w466:dbl)  [unwired: 1 out]
                        n230 = Max & Min(x=50.0, y=w466) -> (min(x,y)=w465:dbl)  [unwired: 1 out]
                        n231 = Build Array(w465) -> (w467:dbl[])
                      }
                    }
                    n232 = Index Array(array=w422, index #1=5 ("index"), index #2=7 ("index"), index #3=6 ("index"), index #4=9 ("index"), index #5=5 ("index")) -> (element #1=w423:dbl, element #2=w439:dbl, element #3=w437:dbl, element #4=w435:dbl, element #5=w431:dbl)
                    n233 = Square(x=w428) -> (x^2=w427:dbl[])
                    n234 = Compound Arithmetic op=MULTIPLY(w427, w437) -> (w433:dbl[])
                    n235 = Compound Arithmetic op=MULTIPLY(w439, w428, w427) -> (w434:dbl[])
                    n236 = Compound Arithmetic op=MULTIPLY(w428, w435) -> (w432:dbl[])
                    n237 = Compound Arithmetic op=ADD(w434, w433, w432, w431) -> (w429:dbl[])
                  }
                  frame #2 {
                    n238 = for {
                      tunnel: [w489] -> w478 mode=indexing
                      tunnel: w483 -> [w493] mode=indexing
                      tunnel: w482 -> [w491] mode=indexing
                      tunnel: [1.0] -> w477 mode=indexing
                      n239 = Square(x=w493) -> (x^2=w496:dbl)
                      n240 = Square(x=w491) -> (x^2=w497:dbl)
                      n241 = Sign(1:w493) -> (0:w492:dbl)
                      n242 = Absolute Value(x=w493) -> (abs(x)=w495:dbl)
                      n243 = Multiply(x=w491, y=w492) -> (x*y=w490:dbl)
                      n244 = Greater Or Equal?(x=w495, y=w491) -> (x >= y?=w494:bool)
                      n245 = Add(x=w496, y=w497) -> (x+y=w498:dbl)
                      n246 = Divide(x=w498, y=w493) -> (x/y=w499:dbl)
                      n247 = Multiply(x=w499, y=0.5) -> (x*y=w501:dbl)
                      n248 = Select(t=w490, s=w494, f=w501) -> (s? t:f=w489:dbl)
                    }
                    n249 = Add Array Elements(numeric array=w477) -> (sum=w476:dbl)
                    n250 = Multiply(x=w478, y="gain(<1)") -> (x*y=w469:dbl[])
                    n251 = Add Array Elements(numeric array=w469) -> (sum=w480:dbl)
                    n252 = global read "rio_Global.vi" "wheel base"() -> (w472:dbl)
                    n253 = Divide(x=w480, y=w476) -> (x/y=w475:dbl)
                    n254 = Divide(x=w472, y=w475) -> (x/y=w474:dbl)
                    n255 = Inverse Tangent(1:w474) -> (0:w484:dbl)
                    n256 = Multiply(x=w484, y=180.0) -> (x*y=w486:dbl)
                    n257 = Divide(x=w486, y=3.141592653589793) -> (x/y=w481:dbl)
                    n258 = global read "rio_Global.vi" "ratio"() -> (w471:dbl)
                    n259 = Multiply(x=w471, y=w481) -> (x*y=w470:dbl)
                    "cmd steer" <- w470
                    n260 = global write "rio_Global.vi" "cmd steer"(w470) -> ()
                  }
                  frame #3 {
                    n261 = global read "rio_Global.vi" "C_mdps str_ang"() -> (w502:dbl)
                    n262 = Subtract(x=w506, y=w502) -> (x-y=w505:dbl)
                    n263 = disable-structure shown="Enabled" {
                      disable-tunnel: [w520 w558] -> w507
                      disable-tunnel: w506 -> [w518 _]
                      disable-tunnel: w505 -> [w512 w553]
                      disable-tunnel: w504 -> [w510 _]
                      disable-tunnel: "Kp" -> [w508 w559]
                      frame Disabled {
                        n264 = Square(x=w512) -> (x^2=w513:dbl)
                        n265 = Absolute Value(x=w512) -> (abs(x)=w511:dbl)
                        n266 = Multiply(x=w513, y=w512) -> (x*y=w515:dbl)
                        n267 = Greater Or Equal?(x=w511, y=1.0) -> (x >= y?=w516:bool)
                        n268 = Select(t=w515, s=w516, f=w512) -> (s? t:f=w514:dbl)
                        n269 = Multiply(x=w514, y=0.002) -> (x*y=w509:dbl)
                        n270 = Multiply(x=w508, y=w509) -> (x*y=w519:dbl)
                        n271 = disable-structure shown="Disabled" {
                          disable-tunnel: [w528 w547] -> w520
                          disable-tunnel: w519 -> [w522 w548]
                          disable-tunnel: w518 -> [_ w538]
                          disable-tunnel: w510 -> [_ w535]
                          frame Disabled {
                            n272 = Absolute Value(x=w522) -> (abs(x)=w527:dbl)
                            n273 = Greater?(x=w527, y="deadzone") -> (0:w526:bool)
                            n274 = Negate(x="visco") -> (-x=w530:dbl)
                            n275 = Select(t=w522, s=w526, f=0.0) -> (s? t:f=w523:dbl)
                            n276 = call "visco.vi"("min"=w530, "max"="visco", "input"=w523) -> ("output"=w528:dbl)  [unwired: 8 in]
                          }
                          frame Enabled {
                            n277 = Square(x=w538) -> (x^2=w539:dbl)
                            n278 = Multiply(x=w539, y=w538) -> (x*y=w537:dbl)
                            n279 = Multiply(x=w535, y="lane center") -> (x*y=w534:dbl)
                            n280 = Multiply(x=0.002 ("y"), y=w537) -> (x*y=w545:dbl)
                            n281 = In Range and Coerce(upper limit=0.2, x=w534, lower limit=-0.2) -> (coerced(x)=w531:dbl)  [unwired: 1 out]
                            n282 = Multiply(x="Kf", y=w545) -> (x*y=w541:dbl)
                            n283 = In Range and Coerce(upper limit=0.35, x=w541, lower limit=-0.35) -> (coerced(x)=w540:dbl)  [unwired: 1 out]
                            n284 = Compound Arithmetic op=ADD(w531, w540, w548) -> (w547:dbl)
                          }
                        }
                      }
                      frame Enabled {
                        n285 = Divide(x=w553, y=3.0) -> (x/y=w551:dbl)
                        n286 = Compound Arithmetic op=MULTIPLY(w551, w551, w551) -> (w550:dbl)
                        n287 = local read "rate limit"() -> (w556:dbl)
                        n288 = Multiply(x=w550, y=0.0001) -> (x*y=w560:dbl)
                        n289 = global read "rio_Global.vi" "steering torque"() -> (w549:dbl)
                        n290 = Multiply(x=w559, y=w560) -> (x*y=w557:dbl)
                        n291 = Negate(x=w556) -> (-x=w555:dbl)
                        n292 = In Range and Coerce(upper limit=w556, x=w557, lower limit=w555) -> (coerced(x)=w554:dbl)  [unwired: 1 out]
                        n293 = Add(x=w554, y=w549) -> (x+y=w558:dbl)
                        "Numeric" <- w553
                      }
                    }
                  }
                }
              }
            }
            n294 = In Range and Coerce(upper limit=0.4, x=w350, lower limit=-0.4) -> (coerced(x)=w335:dbl)  [unwired: 1 out]
            n295 = global write "rio_Global.vi" "Ref_str_torque"(w335) -> ()
          }
          frame #3 {
            n296 = global read "rio_Global.vi" "C_gear selector disp"() -> (w562:u8)
            n297 = global read "rio_Global.vi" "Ref_VS"() -> (w567:dbl)
            n298 = Select(t=w567, s="Velocity input", f="manual speed") -> (s? t:f=w563:dbl)
            n299 = case shown="1" w562 {
              tunnel: [_ w568 w573] -> w564
              tunnel: w563 -> [_ w570 w574]
              frame 0, Default {
                # "P,N"
              }
              frame 1 {
                # "D"
                n300 = Greater Than 0?(x=w570) -> (x > 0?=w571:bool)
                n301 = Select(t=w570, s=w571, f=0.0) -> (s? t:f=w568:dbl)
              }
              frame 2 {
                # "R"
                n302 = Less Than 0?(x=w574) -> (x < 0?=w575:bool)
                n303 = Select(t=w574, s=w575, f=0.0) -> (s? t:f=w573:dbl)
              }
            }
          }
          frame #4 {
            w585 = 3.6  # m/2tokm/h
            w587 = 5.0  # 0.5g
            n304 = global read "rio_Global.vi" "M_headway"() -> (w582:dbl)
            n305 = disable-structure shown="Enabled" {
              disable-tunnel: w576 -> [w597 w628]
              disable-tunnel: [w596 w625] -> w590
              disable-tunnel: [_ w624] -> w577
              frame Disabled {
                n306 = flat-sequence {
                  tunnel: w597 -> [w622]
                  tunnel: [w621] -> w596
                  frame #0 {
                    w604 = dbl[] [0.016, 0.025, 0.08]  # V_PID_gain
                    n307 = global read "rio_Global.vi" "C_VS_CAN"() -> (w598:dbl)
                    n308 = Subtract(x=w622, y=w598) -> (x-y=w623:dbl)
                    n309 = In Range and Coerce(upper limit=20.0, x=w623, lower limit=-999.0) -> (coerced(x)=w600:dbl)  [unwired: 1 out]
                    n310 = feedback #1(w600) -> (w602:dbl)
                    n311 = feedback-in #1(w600) -> ()
                    n312 = Absolute Value(x=w600) -> (abs(x)=w608:dbl)
                    n313 = Multiply(x=w600, y=0.01) -> (x*y=w618:dbl)
                    n314 = Subtract(x=w600, y=w602) -> (x-y=w601:dbl)
                    n315 = Greater?(x=w608, y=1.0) -> (0:w605:bool)
                    n316 = feedback #2(0.0) -> (w617:dbl)
                    n317 = Multiply(x=w617, y=0.95) -> (x*y=w611:dbl)
                    n318 = Add(x=w611, y=w618) -> (x+y=w612:dbl)
                    n319 = feedback-in #2(w612) -> ()
                    n320 = Select(t=w600, s=w605, f=0.0) -> (s? t:f=w615:dbl)
                    n321 = Divide(x=w601, y=0.01) -> (x/y=w599:dbl)
                    n322 = Build Array(w615, w612, w599) -> (w614:dbl[])
                    n323 = Multiply(x=w604, y=w614) -> (x*y=w613:dbl[])
                    n324 = Add Array Elements(numeric array=w613) -> (sum=w621:dbl)
                  }
                }
              }
              frame Enabled {
                n325 = global read "rio_Global.vi" "PWM GAS"() -> (w640:dbl)
                n326 = Subtract(x=w640, y=1000.0) -> (x-y=w637:dbl)
                n327 = global read "rio_Global.vi" "C_VS_CAN"() -> (w624:dbl)
                n328 = Multiply(x=w637, y=0.1) -> (x*y=w626:dbl)
                n329 = Subtract(x=w628, y=w624) -> (x-y=w627:dbl)
                n330 = feedback-in #3(w626) -> ()
                n331 = feedback #3(0.0) -> (w632:dbl)
                n332 = feedback #4(0.0) -> (w630:dbl)
                n333 = feedback-in #4(w624) -> ()
                n334 = Subtract(x=w626, y=w632) -> (x-y=w631:dbl)
                n335 = Equal?(x=w626, y=w632) -> (x = y?=w633:bool)
                n336 = Subtract(x=w624, y=w630) -> (x-y=w629:dbl)
                n337 = Equal?(x=w624, y=w630) -> (x = y?=w634:bool)
                n338 = case shown="False" w634 {
                  tunnel: w633 -> [_ w658]
                  tunnel: w631 -> [w654 _]
                  tunnel: w629 -> [w653 _]
                  tunnel: w627 -> [w652 w656]
                  tunnel: w626 -> [w651 w655]
                  tunnel: [w650 w657] -> w625
                  frame False {
                    n339 = Divide(x=w654, y=w653) -> (x/y=w645:dbl)
                    n340 = Absolute Value(x=w645) -> (abs(x)=w644:dbl)
                    n341 = In Range and Coerce(upper limit="upper limit", x=w644, lower limit=0.01) -> (coerced(x)=w641:dbl)  [unwired: 1 out]
                    n342 = Multiply(x=w652, y=w641) -> (x*y=w647:dbl)
                    n343 = In Range and Coerce(upper limit=25.0, x=w647, lower limit=-25.0) -> (coerced(x)=w646:dbl)  [unwired: 1 out]
                    n344 = Add(x=w651, y=w646) -> (x+y=w650:dbl)
                  }
                  frame True {
                    n345 = case shown="False" w658 {
                      tunnel: [w663 w668] -> w657
                      tunnel: w656 -> [w662 w667]
                      tunnel: w655 -> [w664 w665]
                      frame False {
                        n346 = In Range and Coerce(upper limit=5.0, x=w662, lower limit=-5.0) -> (coerced(x)=w661:dbl)  [unwired: 1 out]
                        n347 = Add(x=w664, y=w661) -> (x+y=w663:dbl)
                      }
                      frame True {
                        n348 = Equal To 0?(x=w667) -> (x = 0?=w666:bool)
                        n349 = case shown="False" w666 {
                          tunnel: w667 -> [w672 _]
                          tunnel: [w669 w673] -> w668
                          tunnel: w665 -> [_ w673]
                          frame False {
                            n350 = In Range and Coerce(upper limit=1.0, x=w672, lower limit=-1.0) -> (coerced(x)=w669:dbl)  [unwired: 1 out]
                          }
                          frame True {
                          }
                        }
                      }
                    }
                  }
                }
              }
            }
            "VS_CAN" <- w577
            n351 = global read "rio_Global.vi" "C_APV"() -> (→"APV":dbl)
            n352 = Multiply(x=w587, y=w582) -> (x*y=w586:dbl)
            n353 = Multiply(x=w585, y=w586) -> (x*y=→"recomammed Speed [km/h]":dbl)
            n354 = Not Equal To 0?(x=w576) -> (x != 0?=w588:bool)
            n355 = global read "rio_Global.vi" "C_MCP"() -> (w581:dbl)
            n356 = global read "rio_Global.vi" "Auto"() -> (w580:bool)
            "Auto" <- w580
            n357 = local read "T out"() -> (w592:i32)
            n358 = local read "T init"() -> (w591:i32)
            n359 = Greater Or Equal?(x=w591, y=w592) -> (x >= y?=w589:bool)
            n360 = Less?(x=w581, y=5.0) -> (x < y?=w594:bool)
            n361 = Compound Arithmetic op=AND(w589, w594, w580, w588) -> (w593:bool)
            n362 = case shown="False" w593 {
              tunnel: [1000.0 ("Numeric") w687] -> w579
              tunnel: w590 -> [_ w693]
              tunnel: w592 -> [w674 _]
              tunnel: [_ TRUE] -> w578
              frame False {
                n363 = local read "T init"() -> (w675:i32)
                n364 = Less Or Equal?(x=w675, y=w674) -> (x <= y?=w676:bool)
                n365 = case shown="True" w676 {
                  tunnel: w674 -> [_ w679]
                  frame False {
                    n366 = local write "T init"(1 ("T init")) -> ()
                  }
                  frame True {
                    n367 = local read "T init"() -> (w682:i32)
                    n368 = Increment(x=w682) -> (x+1=w681:i32)
                    n369 = Max & Min(x=w681, y=w679) -> (min(x,y)=w680:i32)  [unwired: 1 out]
                    n370 = local write "T init"(w680) -> ()
                  }
                }
              }
              frame True {
                w686 = 1000.0 ("x")
                n371 = disable-structure shown="Enabled" {
                  disable-tunnel: [w699 1000.0 ("PWM GAS")] -> w688
                  frame Disabled {
                    n372 = global read "rio_Global.vi" "PWM GAS"() -> (w699:dbl)
                  }
                  frame Enabled {
                  }
                }
                n373 = Multiply(x=10.0, y=w693) -> (x*y=w691:dbl)
                n374 = Add(x=w691, y=w688) -> (x+y=w690:dbl)
                n375 = In Range and Coerce(upper limit=1700.0, x=w690, lower limit=w686) -> (coerced(x)=w687:dbl)  [unwired: 1 out]
                n376 = Subtract(x=w687, y=w686) -> (x-y=w685:dbl)
                n377 = Multiply(x=w685, y=0.1) -> (x*y=w683:dbl)
                n378 = To Long Integer(number=w683) -> (32bit integer=w695:i32)
                n379 = Add(x=w695, y=20) -> (x+y=w697:i32)
                "T out" <- w697
                n380 = Increment(x=w697) -> (x+1=→"T init":i32)
              }
            }
            "PWM GAS" <- w579
            n381 = global write "rio_Global.vi" "Solenoid"(w578) -> ()
            n382 = global write "rio_Global.vi" "PWM GAS"(w579) -> ()
          }
          frame #5 {
            n383 = global read "rio_Global.vi" "C_mdps str_ang"() -> (→"mdps str_ang":dbl)
            n384 = global read "rio_Global.vi" "steering torque"() -> (w705:dbl)
            n385 = global read "rio_Global.vi" "Ref_str_ang"() -> (w701:dbl)
            n386 = global read "rio_Global.vi" "C_mdps torque volt"() -> (w702:dbl)
            n387 = Add(x="rate limit", y=w705) -> (x+y=w712:dbl)
            n388 = Subtract(x=w705, y="rate limit") -> (x-y=w711:dbl)
            n389 = Select(t=w701, s="Steering torque input", f="Manual Steering torque") -> (s? t:f=w707:dbl)
            n390 = In Range and Coerce(upper limit=w712, x=w707, lower limit=w711) -> (coerced(x)=w708:dbl)  [unwired: 1 out]
            n391 = Negate(x=w702) -> (-x=w710:dbl)
            "mdps torque volt" <- w710
            n392 = global read "rio_Global.vi" "Auto"() -> (w703:bool)
            n393 = Merge Signals(w707, w710) -> (→"Waveform Chart":dynamicdata)
            n394 = Select(t=w708, s=w703, f=0.0) -> (s? t:f=w704:dbl)
            n395 = global write "rio_Global.vi" "steering torque"(w704) -> ()
          }
        }
      }
    }
  }
  n396 = flat-sequence {
    tunnel: [w717] -> w1
    tunnel: w1 -> [w724]
    frame #0 {
      n397 = for {
        N: 257 -> [_]
        tunnel: [w723] -> w721 mode=indexing
        i -> [w723]
      }
      n398 = Multiply(x=w721, y=0.5) -> (x*y=w717:dbl[])
      n399 = Array Subset(array=w717, index=30) -> (w718:dbl[])  [unwired: 1 in]
      n400 = global write "rio_Global.vi" "x_view"(w718) -> ()
    }
    frame #1 {
      n401 = while {
        tunnel: w724 -> [w725]
        stop <- FALSE stop-if-true
        n402 = flat-sequence {
          tunnel: [w728] -> w726
          tunnel: w725 -> [w728]
          tunnel: w726 -> [w730]
          frame #0 {
            n403 = Wait Until Next ms Multiple(millisecond multiple=u32 33) -> ()  [unwired: 1 out]
          }
          frame #1 {
            n404 = call "mobileye_disp.vi"("x_view"=w730) -> ("XY Graph"=→"XY Graph":cluster{"Y":dbl[], "Y":dbl[]}[])  [unwired: 10 in]
          }
        }
      }
    }
  }
  n405 = disable-structure shown="Enabled" {
    frame Enabled {
      n406 = flat-sequence {
        tunnel: [dbl[] [0.0, 0.0, 0.0, 0.0, 0.0] ("pos(i)")] -> w732
        tunnel: w732 -> [w742]
        frame #0 {
          w735 = FALSE ("get heading")
          w736 = u64 1
          w733 = 0.0 ("dh_hat")
          w739 = 4 ("map")
          n407 = local write "GPS init"(w735) -> ()
          n408 = call "getecefdcmref.vi"("map"=w739) -> ("XYZ"=→"ecef ref":dbl[])  [unwired: 10 in, 4 out]
          "map" <- w739
          "vgain" <- 1.0 ("initH")
          "vcount" <- w736
          "hbias" <- w733
          "hcount" <- w736
          "get heading" <- w735
          "get position" <- w735
          "heading error" <- w733
          "h_gps" <- w733
          "rt" <- w733
          "pos error" <- w733
          "POS init" <- TRUE ("POS init")
        }
        frame #1 {
          n409 = flat-sequence {
            tunnel: [w1199] -> w741
            tunnel: w741 -> [w1207]
            frame #0 {
              n410 = while {
                shift-right: [w1205] -> w1201
                shift-left: refnum<visa-resource-name> "ASRL3::INSTR" ("VISA resource name") -> [w1206]
                stop <- w1204 continue-if-true
                n411 = VISA Open(VISA resource name=w1206) -> (VISA resource name=w1205:refnum<visa-resource-name>, error out=w1204:errorcluster)  [unwired: 4 in]
              }
              n412 = VISA Clear(VISA resource name=w1201) -> (VISA resource name out=w1203:refnum<visa-resource-name>)  [unwired: 1 in, 1 out]
              n413 = property class="Instr"(reference=w1203, "General Settings:Timeout Value"=u32 10) -> (reference out=w1199:refnum<visa-resource-name>)  [unwired: 1 in, 1 out]
            }
            frame #1 {
              n414 = while {
                tunnel: w1207 -> [w1208]
                stop <- FALSE stop-if-true
                n415 = flat-sequence {
                  tunnel: w1208 -> [w1210]
                  frame #0 {
                    n416 = VISA Read(VISA resource name=w1210, byte count=u32 100) -> (read buffer=w1211:string)  [unwired: 1 in, 3 out]
                    n417 = case shown="Default" w1211 {
                      selector: w1211 -> [_ w1213]
                      frame "" {
                      }
                      frame Default {
                        n418 = local read "ecef ref"() -> (w1214:dbl[])
                        n419 = call "nmea.vi"("ecef ref"=w1214, "NMEA"=w1213) -> ("output"=w1216:dbl[], "type"=w1215:u32)  [unwired: 8 in]
                        n420 = case shown="2" w1215 {
                          tunnel: w1216 -> [_ w1217 w1252]
                          frame 0, Default {
                          }
                          frame 1 {
                            n421 = global write "rio_Global.vi" "gps_pos 1"(w1217) -> ()
                            n422 = disable-structure shown="Enabled" {
                              disable-tunnel: w1217 -> [w1219 _]
                              frame Enabled {
                                n423 = Index Array(array=w1219, index=1) -> (element=w1221:dbl)
                                n424 = Not Equal To 0?(x=w1221) -> (x != 0?=w1218:bool)
                                n425 = case shown="True" w1218 {
                                tunnel: w1219 -> [_ w1241]
                                frame False {
                                }
                                frame True {
                                n426 = Get Date/Time In Seconds() -> (seconds since 1Jan1904=w1226:timestamp)
                                n427 = global read "rio_Global.vi" "LCM_GGA_T"() -> (w1250:T23)
                                n428 = To Double Precision Float(number=w1226) -> (double precision float=w1225:dbl)
                                n429 = Array To Cluster(array=w1241) -> (cluster=w1249:T24)
                                n430 = Unbundle By Name(w1250) -> ("hash"=w1246:i64)
                                n431 = Multiply(x=w1225, y=1000000.0) -> (x*y=w1223:dbl)
                                n432 = Unbundle(w1249) -> ("output[0]"=w1251:dbl, "output[2]"=w1240:dbl, "output[3]"=w1239:dbl, "output[4]"=w1238:dbl, "output[6]"=w1237:dbl, "output[7]"=w1235:dbl, "output[8]"=w1233:dbl, "output[9]"=w1231:dbl, "output[12]"=w1230:dbl, "output[13]"=w1229:dbl, "output[14]"=w1228:dbl)  [unwired: 4 out]
                                n433 = call "hash.vi"("input"=w1246) -> ("output"=w1245:i64)  [unwired: 10 in]
                                n434 = To Quad Integer(1:w1223) -> (0:w1222:i64)
                                n435 = To Long Integer(number=w1237) -> (32bit integer=w1236:i32)
                                n436 = To Long Integer(number=w1235) -> (32bit integer=w1234:i32)
                                n437 = To Long Integer(number=w1233) -> (32bit integer=w1232:i32)
                                n438 = local read "map"() -> (w1227:i32)
                                n439 = Bundle(cluster=w1250, "hash"=w1245, "sys time"=w1222, "time"=w1251, "x"=w1240, "y"=w1239, "h"=w1238, "numSV"=w1236, "postype"=w1234, "lag"=w1232, "hordev"=w1231, "lat"=w1230, "lon"=w1229, "hgt"=w1228, "map_idx"=w1227) -> (w1247:T23)
                                n440 = Flatten To String(anything=w1247, prepend array or string size? (T)=FALSE) -> (data string=w1243:string)  [unwired: 2 in, 2 out]
                                n441 = global read "rio_Global.vi" "LCM"() -> (w1242:T5)
                                n442 = call "LCM_send.vi"("DATA"=w1243, "ID"="GGA_1", "LCM"=w1242) -> ()  [unwired: 6 in, 3 out]
                                }
                                }
                              }
                              frame Disabled {
                              }
                            }
                          }
                          frame 2 {
                            n443 = global write "rio_Global.vi" "gps_vel 1"(w1252) -> ()
                            n444 = disable-structure shown="Enabled" {
                              disable-tunnel: w1252 -> [w1256 _]
                              frame Enabled {
                                n445 = Index Array(array=w1256, index=1) -> (element=w1255:dbl)
                                n446 = Not Equal To 0?(x=w1255) -> (x != 0?=w1253:bool)
                                n447 = case shown="True" w1253 {
                                tunnel: w1256 -> [_ w1275]
                                frame False {
                                }
                                frame True {
                                n448 = Get Date/Time In Seconds() -> (seconds since 1Jan1904=w1261:timestamp)
                                n449 = global read "rio_Global.vi" "LCM_RMC_T"() -> (w1276:T25)
                                n450 = To Double Precision Float(number=w1261) -> (double precision float=w1260:dbl)
                                n451 = Unbundle By Name(w1276) -> ("hash"=w1272:i64)
                                n452 = Multiply(x=w1260, y=1000000.0) -> (x*y=w1258:dbl)
                                n453 = Array To Cluster(array=w1275) -> (cluster=w1274:T26)
                                n454 = call "hash.vi"("input"=w1272) -> ("output"=w1271:i64)  [unwired: 10 in]
                                n455 = To Quad Integer(1:w1258) -> (0:w1257:i64)
                                n456 = Unbundle(w1274) -> ("output[0]"=w1266:dbl, "output[2]"=w1265:dbl, "output[4]"=w1264:dbl, "output[5]"=w1263:dbl, "output[6]"=w1262:dbl)  [unwired: 2 out]
                                n457 = Bundle(cluster=w1276, "hash"=w1271, "sys time"=w1257, "time"=w1266, "speed"=w1265, "heading"=w1264, "lat"=w1263, "lon"=w1262) -> (w1267:T25)
                                n458 = Flatten To String(anything=w1267, prepend array or string size? (T)=FALSE) -> (data string=w1269:string)  [unwired: 2 in, 2 out]
                                n459 = global read "rio_Global.vi" "LCM"() -> (w1268:T5)
                                n460 = call "LCM_send.vi"("DATA"=w1269, "ID"="RMC_1", "LCM"=w1268) -> ()  [unwired: 6 in, 3 out]
                                }
                                }
                              }
                              frame Disabled {
                              }
                            }
                          }
                        }
                      }
                    }
                  }
                }
              }
            }
          }
          n461 = disable-structure shown="Enabled" {
            disable-tunnel: w742 -> [w743 _]
            frame Enabled {
              n462 = while {
                shift-right: [w744] -> _
                shift-left: w743 -> [w745]
                stop <- FALSE stop-if-true
                n463 = flat-sequence {
                  tunnel: [w756] -> w748
                  tunnel: w745 -> [w756]
                  tunnel: w748 -> [w759]
                  tunnel: [w758] -> w747
                  tunnel: [w758] -> w746
                  tunnel: [w1172] -> w744
                  tunnel: w747 -> [w1173]
                  tunnel: w746 -> [w1172]
                  frame #0 {
                    n464 = global read "rio_Global.vi" "C_ts"() -> (→"dt":dbl)
                    n465 = Wait Until Next ms Multiple(millisecond multiple=u32 10) -> (millisecond timer value=w754:u32)
                    n466 = feedback #5(w754) -> (w753:u32)
                    n467 = feedback-in #5(w754) -> ()
                    n468 = Subtract(x=w754, y=w753) -> (x-y=w752:u32)
                    n469 = To Long Integer(number=w752) -> (32bit integer=→"Pos_time 10":i32)
                  }
                  frame #1 {
                    n470 = flat-sequence {
                      tunnel: w759 -> [w766]
                      tunnel: [w766] -> w757
                      tunnel: [w889] -> w758
                      tunnel: w757 -> [w890]
                      frame #0 {
                        n471 = disable-structure shown="Enabled" {
                          disable-tunnel: [w786 w787] -> w761
                          disable-tunnel: [w767 w788] -> w760
                          frame Disabled {
                            n472 = global read "rio_Global.vi" "gps_pos 1"() -> (w783:dbl[])
                            n473 = global read "rio_Global.vi" "gps_pos 2"() -> (w770:dbl[])
                            n474 = Add(x=w783, y=w770) -> (x+y=w785:dbl[])
                            n475 = Index Array(array=w783, index #1=0 ("index")) -> (element #1=w782:dbl, element #2=w781:dbl)  [unwired: 1 in]
                            n476 = Index Array(array=w770, index #1=0 ("index")) -> (element #1=w771:dbl, element #2=w772:dbl)  [unwired: 1 in]
                            n477 = feedback #6(w782) -> (w780:dbl)
                            n478 = feedback-in #6(w782) -> ()
                            n479 = feedback #7(w771) -> (w773:dbl)
                            n480 = feedback-in #7(w771) -> ()
                            n481 = Not Equal?(x=w782, y=w780) -> (x != y?=w779:bool)
                            n482 = Not Equal?(x=w771, y=w773) -> (x != y?=w774:bool)
                            n483 = Not Equal To 0?(x=w781) -> (x != 0?=w778:bool)
                            n484 = Not Equal To 0?(x=w772) -> (x != 0?=w775:bool)
                            n485 = And(x=w779, y=w778) -> (x .and. y?=w768:bool)
                            n486 = And(x=w774, y=w775) -> (x .and. y?=w769:bool)
                            n487 = And(x=w768, y=w769) -> (x .and. y?=w786:bool)
                            n488 = Multiply(x=w785, y=0.5) -> (x*y=w767:dbl[])
                          }
                          frame Enabled {
                            n489 = global read "rio_Global.vi" "gps_pos 1"() -> (w788:dbl[])
                            n490 = Index Array(array=w788, index #1=0 ("index")) -> (element #1=w794:dbl, element #2=w793:dbl)  [unwired: 1 in]
                            n491 = feedback #8(w794) -> (w792:dbl)
                            n492 = feedback-in #8(w794) -> ()
                            n493 = Not Equal?(x=w794, y=w792) -> (x != y?=w791:bool)
                            n494 = Not Equal To 0?(x=w793) -> (x != 0?=w790:bool)
                            n495 = And(x=w791, y=w790) -> (x .and. y?=w787:bool)
                          }
                        }
                        "pos_gps" <- w760
                        n496 = disable-structure shown="Enabled" {
                          disable-tunnel: [w840 w871] -> w765
                          disable-tunnel: [w839 w850] -> w764
                          disable-tunnel: [w811 w861] -> w763
                          disable-tunnel: [w799 w856] -> w762
                          frame Disabled {
                            n497 = global read "rio_Global.vi" "gps_vel 1"() -> (w838:dbl[])
                            n498 = global read "rio_Global.vi" "gps_vel 2"() -> (w817:dbl[])
                            n499 = Index Array(array=w838, index #1=0 ("index"), index #2=1 ("index"), index #3=4 ("index"), index #4=2 ("index")) -> (element #1=w829:dbl, element #2=w834:dbl, element #3=w831:dbl, element #4=w803:dbl)
                            n500 = Index Array(array=w817, index #1=0 ("index"), index #2=1 ("index"), index #3=4 ("index"), index #4=2 ("index")) -> (element #1=w826:dbl, element #2=w821:dbl, element #3=w824:dbl, element #4=w802:dbl)
                            n501 = global read "rio_Global.vi" "C_VS_CAN"() -> (w796:dbl)
                            n502 = global read "rio_Global.vi" "C_VS_CAN"() -> (w843:dbl)
                            n503 = Add(x=w803, y=w802) -> (x+y=w801:dbl)
                            n504 = Not Equal To 0?(x=w821) -> (x != 0?=w822:bool)
                            n505 = call "angleconv.vi"("deg"=w831) -> ("rad"=w814:dbl)  [unwired: 9 in, 1 out]
                            n506 = call "angleconv.vi"("deg"=w824) -> ("rad"=w813:dbl)  [unwired: 9 in, 1 out]
                            n507 = feedback #9(0.0 ("Real Matrix Element")) -> (w828:dbl)
                            n508 = feedback-in #9(w829) -> ()
                            n509 = feedback #10(0.0 ("Real Matrix Element")) -> (w827:dbl)
                            n510 = feedback-in #10(w826) -> ()
                            n511 = Not Equal?(x=w829, y=w828) -> (x != y?=w835:bool)
                            n512 = Not Equal?(x=w826, y=w827) -> (x != y?=w820:bool)
                            n513 = Not Equal To 0?(x=w834) -> (x != 0?=w833:bool)
                            n514 = Greater Or Equal To 0?(x=w843) -> (x >= 0?=w844:bool)
                            n515 = Absolute Value(x=w796) -> (abs(x)=w795:dbl)
                            n516 = Multiply(x=w801, y=0.5) -> (x*y=w810:dbl)
                            n517 = call "headingweightsum.vi"("a"=0.5, "h1"=w813, "h2"=w814) -> ("a*h2+(1-a)*h1"=w842:dbl)  [unwired: 8 in]
                            n518 = And(x=w835, y=w833) -> (x .and. y?=w816:bool)
                            n519 = And(x=w820, y=w822) -> (x .and. y?=w815:bool)
                            n520 = Divide(x=w810, y=w795) -> (x/y=w811:dbl)
                            n521 = Select(t=0.0, s=w844, f=3.141592653589793) -> (s? t:f=w841:dbl)
                            n522 = Decrement(x=w811) -> (x-1=w807:dbl)
                            n523 = call "headingoperater.vi"("h1"=w841, "h2"=w842) -> ("h2-h1"=w840:dbl)  [unwired: 8 in, 1 out]
                            n524 = And(x=w816, y=w815) -> (x .and. y?=w839:bool)
                            n525 = Absolute Value(x=w807) -> (abs(x)=w808:dbl)
                            n526 = Greater?(x=w795, y=15.0) -> (0:w797:bool)
                            n527 = Less?(x=w808, y=0.05) -> (x < y?=w800:bool)
                            n528 = Compound Arithmetic op=AND(w797, w800, w839) -> (w799:bool)
                          }
                          frame Enabled {
                            n529 = global read "rio_Global.vi" "gps_vel 1"() -> (w870:dbl[])
                            n530 = global read "rio_Global.vi" "C_VS_CAN"() -> (w854:dbl)
                            n531 = global read "rio_Global.vi" "C_VS_CAN"() -> (w873:dbl)
                            n532 = Index Array(array=w870, index #1=0 ("index"), index #2=1 ("index"), index #3=4 ("index"), index #4=2 ("index")) -> (element #1=w849:dbl, element #2=w866:dbl, element #3=w863:dbl, element #4=w852:dbl)
                            n533 = Greater Or Equal To 0?(x=w873) -> (x >= 0?=w874:bool)
                            n534 = Absolute Value(x=w854) -> (abs(x)=w853:dbl)
                            n535 = feedback #11(w849) -> (w862:dbl)
                            n536 = feedback-in #11(w849) -> ()
                            n537 = Divide(x=w852, y=w853) -> (x/y=w861:dbl)
                            n538 = call "angleconv.vi"("deg"=w863) -> ("rad"=w851:dbl)  [unwired: 9 in, 1 out]
                            n539 = Select(t=0.0, s=w874, f=3.141592653589793) -> (s? t:f=w872:dbl)
                            n540 = Not Equal?(x=w849, y=w862) -> (x != y?=w867:bool)
                            n541 = Not Equal To 0?(x=w866) -> (x != 0?=w865:bool)
                            n542 = Decrement(x=w861) -> (x-1=w858:dbl)
                            n543 = call "headingoperater.vi"("h1"=w872, "h2"=w851) -> ("h2-h1"=w871:dbl)  [unwired: 8 in, 1 out]
                            n544 = And(x=w867, y=w865) -> (x .and. y?=w850:bool)
                            n545 = Absolute Value(x=w858) -> (abs(x)=w859:dbl)
                            n546 = Greater?(x=w853, y=15.0) -> (0:w847:bool)
                            n547 = Less?(x=w859, y=0.05) -> (x < y?=w848:bool)
                            n548 = Compound Arithmetic op=AND(w850, w848, w847) -> (w856:bool)
                          }
                        }
                        n549 = local write "get position"(w761) -> ()
                        n550 = local write "h_gps"(w765) -> ()
                        n551 = local write "get heading"(w764) -> ()
                        n552 = case shown="True" w762 {
                          tunnel: w763 -> [_ w884]
                          frame False {
                          }
                          frame True {
                            w878 = u64 18446744073709551615
                            n553 = local read "vcount"() -> (w881:u64)
                            n554 = local read "vgain"() -> (w886:dbl)
                            n555 = Increment(x=w881) -> (x+1=w880:u64)
                            n556 = Not Equal?(x=w881, y=w878) -> (x != y?=w879:bool)
                            n557 = Multiply(x=w886, y=w881) -> (x*y=w885:dbl)
                            n558 = Add(x=w884, y=w885) -> (x+y=w883:dbl)
                            n559 = Select(t=w880, s=w879, f=w878) -> (s? t:f=w877:u64)
                            n560 = local write "vcount"(w877) -> ()
                            n561 = Divide(x=w883, y=w877) -> (x/y=w882:dbl)
                            n562 = local write "vgain"(w882) -> ()
                          }
                        }
                      }
                      frame #1 {
                        n563 = local read "dt"() -> (w888:dbl)
                        n564 = Greater Than 0?(x=w888) -> (x > 0?=w887:bool)
                        n565 = case shown="True" w887 {
                          tunnel: w890 -> [w891 w894]
                          tunnel: [w891 w893] -> w889
                          frame False {
                          }
                          frame True {
                            n566 = flat-sequence {
                              tunnel: w894 -> [w928]
                              tunnel: [w906] -> w892
                              tunnel: [w956] -> w893
                              tunnel: w892 -> [w955]
                              frame #0 {
                                n567 = global read "rio_Global.vi" "C_VS_CAN"() -> (w896:dbl)
                                n568 = Equal To 0?(x=w896) -> (x = 0?=w898:bool)
                                n569 = case shown="True" w898 {
                                tunnel: [w930 _] -> w897
                                frame False {
                                n570 = global read "rio_Global.vi" "C_yaw_rate"() -> (w929:dbl)
                                n571 = local read "hbias"() -> (w933:dbl)
                                n572 = Subtract(x=w929, y=w933) -> (x-y=w931:dbl)
                                n573 = Negate(x=w931) -> (-x=w932:dbl)
                                n574 = call "angleconv.vi"("deg"=w932) -> ("rad"=w930:dbl)  [unwired: 9 in, 1 out]
                                }
                                frame True {
                                w937 = u64 18446744073709551615
                                n575 = local read "hcount"() -> (w940:u64)
                                n576 = local read "hbias"() -> (w943:dbl)
                                n577 = Increment(x=w940) -> (x+1=w939:u64)
                                n578 = global read "rio_Global.vi" "C_yaw_rate"() -> (w934:dbl)
                                n579 = Not Equal?(x=w940, y=w937) -> (x != y?=w938:bool)
                                n580 = Multiply(x=w943, y=w940) -> (x*y=w942:dbl)
                                n581 = Add(x=w934, y=w942) -> (x+y=w941:dbl)
                                n582 = Select(t=w939, s=w938, f=w937) -> (s? t:f=w936:u64)
                                n583 = local write "hcount"(w936) -> ()
                                n584 = Divide(x=w941, y=w936) -> (x/y=w935:dbl)
                                n585 = local write "hbias"(w935) -> ()
                                }
                                }
                                n586 = global read "rio_Global.vi" "C_VS_CAN"() -> (w895:dbl)
                                n587 = local read "vgain"() -> (w901:dbl)
                                n588 = Multiply(x=w895, y=w901) -> (x*y=w900:dbl)
                                n589 = Divide(x=w900, y=3.6) -> (x/y=w899:dbl)
                                n590 = Index Array(array=w928, index #1=0 ("index"), index #2=3 ("index"), index #3=1 ("index"), index #4=3 ("index")) -> (element #1=w922:dbl, element #2=w920:dbl, element #3=w916:dbl, element #4=w911:dbl)
                                n591 = local read "dt"() -> (w925:dbl)
                                n592 = local read "dt"() -> (w909:dbl)
                                n593 = Multiply(x=w899, y=w925) -> (x*y=w921:dbl)
                                n594 = Multiply(x=w909, y=w897) -> (x*y=w902:dbl)
                                n595 = Cosine(x=w920) -> (cos(x)=w926:dbl)
                                n596 = Sine(x=w920) -> (sin(x)=w919:dbl)
                                n597 = Multiply(x=w926, y=w921) -> (x*y=w923:dbl)
                                n598 = Multiply(x=w921, y=w919) -> (x*y=w918:dbl)
                                n599 = local write "rt"(w902) -> ()
                                n600 = Add(x=w922, y=w923) -> (x+y=w915:dbl)
                                n601 = Add(x=w918, y=w916) -> (x+y=w914:dbl)
                                n602 = call "headingoperater.vi"("h1"=w902, "h2"=w911) -> ("h2+h1"=w910:dbl)  [unwired: 8 in, 1 out]
                                n603 = Build Array(w915, w914, w899, w910, w897) -> (w906:dbl[])
                                n604 = Index Array(array=w906, index=3) -> (element=w905:dbl)
                                n605 = local read "h_gps"() -> (w904:dbl)
                                n606 = call "headingoperater.vi"("h1"=w905, "h2"=w904) -> ("h2-h1"=w908:dbl)  [unwired: 8 in, 1 out]
                                n607 = Absolute Value(x=w908) -> (abs(x)=w903:dbl)
                                n608 = local write "heading error"(w903) -> ()
                              }
                              frame #1 {
                                n609 = local read "get heading"() -> (w963:bool)
                                n610 = local read "get position"() -> (w962:bool)
                                n611 = local read "POS init"() -> (w948:bool)
                                n612 = case shown="False" w948 {
                                tunnel: w963 -> [w966 w973]
                                tunnel: w962 -> [w970 w972]
                                tunnel: [w964 w971] -> w958
                                frame False {
                                n613 = local read "heading error"() -> (w967:dbl)
                                n614 = Less?(x=w967, y=0.05) -> (x < y?=w968:bool)
                                n615 = And(x=w966, y=w968) -> (x .and. y?=w965:bool)
                                n616 = Or(x=w965, y=w970) -> (x .or. y?=w964:bool)
                                }
                                frame True {
                                n617 = disable-structure shown="Enabled" {
                                disable-tunnel: w973 -> [w976 w978]
                                disable-tunnel: w972 -> [w975 w977]
                                disable-tunnel: [w974 w979] -> w971
                                frame Disabled {
                                n618 = And(x=w976, y=w975) -> (x .and. y?=w974:bool)
                                }
                                frame Enabled {
                                n619 = Or(x=w978, y=w977) -> (x .or. y?=w979:bool)
                                }
                                }
                                }
                                }
                                n620 = global read "rio_Global.vi" "C_VS_CAN"() -> (w961:dbl)
                                n621 = local read "heading error"() -> (w951:dbl)
                                n622 = Absolute Value(x=w961) -> (abs(x)=w960:dbl)
                                n623 = local read "POS init"() -> (w949:bool)
                                n624 = Greater?(x=w960, y=5.0) -> (0:w957:bool)
                                n625 = Less?(x=w951, y=1.0) -> (x < y?=w950:bool)
                                n626 = Or(x=w950, y=w949) -> (x .or. y?=w952:bool)
                                n627 = And(x=w958, y=w957) -> (x .and. y?=w953:bool)
                                n628 = And(x=w953, y=w952) -> (x .and. y?=w946:bool)
                                n629 = Select(t=FALSE, s="GPS init", f=w946) -> (s? t:f=w945:bool)
                                n630 = case shown="True" w945 {
                                tunnel: [w983 w1012] -> w956
                                tunnel: w955 -> [w984 w1015]
                                frame False {
                                n631 = global read "rio_Global.vi" "C_VS_CAN"() -> (w987:dbl)
                                n632 = local read "POS init"() -> (w986:bool)
                                n633 = Equal To 0?(x=w987) -> (x = 0?=w985:bool)
                                n634 = local read "GPS init"() -> (w980:bool)
                                n635 = And(x=w986, y=w985) -> (x .and. y?=w982:bool)
                                n636 = Or(x=w982, y=w980) -> (x .or. y?=w981:bool)
                                n637 = case shown="True" w981 {
                                tunnel: w984 -> [w988 w989]
                                tunnel: [w988 w991] -> w983
                                tunnel: w980 -> [_ w990]
                                frame False {
                                }
                                frame True {
                                n638 = case shown="False" w990 {
                                tunnel: [w1002 w1011] -> w991
                                tunnel: w989 -> [w997 w1005]
                                frame True {
                                n639 = Index Array(array=w997, index #1=2 ("index")) -> (element #2=w992:dbl, element #3=w995:dbl)  [unwired: 2 in, 1 out]
                                n640 = local read "pos_gps"() -> (w998:dbl[])
                                n641 = local write "GPS init"(FALSE ("GPS init")) -> ()
                                n642 = Index Array(array=w998, index #1=2 ("index")) -> (element #1=w1000:dbl, element #2=w999:dbl)  [unwired: 1 in]
                                n643 = local read "h_gps"() -> (w993:dbl)
                                n644 = Build Array(w1000, w999, w992, w993, w995) -> (w1002:dbl[])
                                }
                                frame False {
                                w1004 = 0.0 ("element")
                                n645 = Index Array(array=w1005, index=3) -> (element=w1003:dbl)
                                n646 = local read "pos_gps"() -> (w1007:dbl[])
                                n647 = Index Array(array=w1007, index #1=2 ("index")) -> (element #1=w1009:dbl, element #2=w1008:dbl)  [unwired: 1 in]
                                n648 = Build Array(w1009, w1008, w1004, w1003, w1004) -> (w1011:dbl[])
                                }
                                }
                                }
                                }
                                }
                                frame True {
                                n649 = flat-sequence {
                                tunnel: w1015 -> [w1016]
                                tunnel: [w1016] -> w1014
                                tunnel: w1014 -> [w1057]
                                tunnel: [w1057] -> w1013
                                tunnel: w1013 -> [w1084]
                                tunnel: [w1088] -> w1012
                                frame #0 {
                                w1025 = 0.0 ("element")
                                w1029 = 0.0 ("element")
                                w1031 = 0.0 ("element")
                                w1033 = 0.0 ("element")
                                w1035 = 0.0 ("element")
                                n650 = Index Array(array=w1016, index #1=3 ("index"), index #2=2 ("index"), index #3=3 ("index"), index #4=2 ("index")) -> (element #1=w1045:dbl, element #2=w1047:dbl, element #3=w1050:dbl, element #4=w1039:dbl)
                                n651 = Negate(x=w1047) -> (-x=w1046:dbl)
                                n652 = Sine & Cosine(0:w1050) -> (1:w1042:dbl, 2:w1040:dbl)
                                n653 = Multiply(x=w1046, y=w1042) -> (x*y=w1043:dbl)
                                n654 = Multiply(x=w1040, y=w1039) -> (x*y=w1038:dbl)
                                n655 = Cosine(x=w1045) -> (cos(x)=w1044:dbl)
                                n656 = Build Array(w1035, w1035, w1044, w1043, 0.0 ("element")) -> (w1037:dbl[])
                                n657 = Build Array(w1033, w1033, w1042, w1038, 0.0 ("element")) -> (w1036:dbl[])
                                n658 = Build Array(w1031, w1031, w1031, w1031, w1031) -> (w1030:dbl[])
                                n659 = Build Array(w1029, w1029, w1029, w1029, 1.0 ("element")) -> (w1027:dbl[])
                                n660 = Build Array(w1025, w1025, w1025, w1025, w1025) -> (w1026:dbl[])
                                n661 = Build Array(w1037, w1036, w1030, w1027, w1026) -> (w1023:dbl[][])
                                n662 = call-poly <vilib>:"Array To Matrix.vi"("Real 2D Array"=w1023) -> ("Real Matrix"=w1021:T27)
                                n663 = global read "rio_Global.vi" "P"() -> (w1024:T27)
                                n664 = Transpose Matrix(1:w1021) -> (0:w1020:T27)
                                n665 = call-poly <vilib>:"Multiply.vi"("Real Matrix B"=w1024, "Real Matrix A"=w1021) -> ("A * B"=w1022:T27)
                                n666 = call-poly <vilib>:"Multiply.vi"("Real Matrix B"=w1020, "Real Matrix A"=w1022) -> ("A * B"=w1019:T27)
                                n667 = global read "rio_Global.vi" "Q"() -> (w1018:T27)
                                n668 = call-poly <vilib>:"Add.vi"("Real Matrix B"=w1018, "Real Matrix A"=w1019) -> ("A + B"=w1017:T27)
                                n669 = global write "rio_Global.vi" "Pp"(w1017) -> ()
                                }
                                frame #1 {
                                n670 = global read "rio_Global.vi" "Pp"() -> (w1082:T27)
                                n671 = global read "rio_Global.vi" "H"() -> (w1081:T27)
                                n672 = Array Subset(array=w1057, index=0, length=2) -> (w1064:dbl[])
                                n673 = local read "pos_gps"() -> (w1060:dbl[])
                                n674 = call-poly <vilib>:"Multiply.vi"("Real Matrix B"=w1082, "Real Matrix A"=w1081) -> ("A * B"=w1080:T27)
                                n675 = Transpose Matrix(1:w1081) -> (0:w1079:T27)
                                n676 = call-poly <vilib>:"Multiply.vi"("Real Matrix B"=w1079, "Real Matrix A"=w1080) -> ("A * B"=w1078:T27)
                                n677 = Array Subset(array=w1060, index=2, length=2) -> (w1063:dbl[])
                                n678 = Subtract(x=w1063, y=w1064) -> (x-y=w1065:dbl[])
                                n679 = global read "rio_Global.vi" "H"() -> (w1076:T27)
                                n680 = global read "rio_Global.vi" "R"() -> (w1077:T27)
                                n681 = global read "rio_Global.vi" "Pp"() -> (w1075:T27)
                                n682 = call-poly <vilib>:"Add.vi"("Real Matrix B"=w1077, "Real Matrix A"=w1078) -> ("A + B"=w1072:T27)
                                n683 = Square(x=w1065) -> (x^2=w1066:dbl[])
                                n684 = Transpose Matrix(1:w1076) -> (0:w1074:T27)
                                n685 = local read "heading error"() -> (w1069:dbl)
                                n686 = call-poly <vilib>:"Multiply.vi"("Real Matrix B"=w1074, "Real Matrix A"=w1075) -> ("A * B"=w1073:T27)
                                n687 = Add Array Elements(numeric array=w1066) -> (sum=w1067:dbl)
                                n688 = call-poly <vilib>:"Inverse Matrix.vi"("Input Matrix"=w1072) -> ("Inverse Matrix"=w1071:T27)  [unwired: 1 in, 1 out]
                                n689 = call-poly <vilib>:"Multiply.vi"("Real Matrix B"=w1071, "Real Matrix A"=w1073) -> ("A * B"=w1070:T27)
                                n690 = Square Root(x=w1067) -> (sqrt(x)=w1056:dbl)
                                n691 = global write "rio_Global.vi" "K"(w1070) -> ()
                                n692 = Less?(x=w1056, y=2.5) -> (x < y?=w1053:bool)
                                n693 = Less?(x=w1069, y=0.05) -> (x < y?=w1054:bool)
                                n694 = And(x=w1054, y=w1053) -> (x .and. y?=w1052:bool)
                                n695 = case shown="True" w1052 {
                                frame False {
                                }
                                frame True {
                                n696 = local write "POS init"(FALSE ("Kalman init")) -> ()
                                }
                                }
                                }
                                frame #2 {
                                n697 = disable-structure shown="Enabled" {
                                disable-tunnel: [w1100 w1101] -> w1087
                                frame Disabled {
                                n698 = local read "get heading"() -> (w1100:bool)
                                }
                                frame Enabled {
                                n699 = local read "heading error"() -> (w1104:dbl)
                                n700 = local read "POS init"() -> (w1102:bool)
                                n701 = Less?(x=w1104, y=0.1) -> (x < y?=w1103:bool)
                                n702 = Or(x=w1103, y=w1102) -> (x .or. y?=w1101:bool)
                                }
                                }
                                n703 = disable-structure shown="Enabled" {
                                disable-tunnel: [w1106 w1108] -> w1086
                                disable-tunnel: w1084 -> [_ w1117]
                                frame Disabled {
                                n704 = local read "get position"() -> (w1106:bool)
                                }
                                frame Enabled {
                                n705 = Array Subset(array=w1117, index=0, length=2) -> (w1115:dbl[])
                                n706 = local read "pos_gps"() -> (w1120:dbl[])
                                n707 = Array Subset(array=w1120, index=2, length=2) -> (w1116:dbl[])
                                n708 = disable-structure shown="Enabled" {
                                disable-tunnel: [w1123 TRUE ("Kalman init")] -> w1110
                                frame Disabled {
                                n709 = local read "POS init"() -> (w1123:bool)
                                }
                                frame Enabled {
                                }
                                }
                                n710 = Subtract(x=w1116, y=w1115) -> (x-y=w1114:dbl[])
                                n711 = Square(x=w1114) -> (x^2=w1113:dbl[])
                                n712 = Add Array Elements(numeric array=w1113) -> (sum=w1112:dbl)
                                n713 = Square Root(x=w1112) -> (sqrt(x)=w1107:dbl)
                                n714 = local write "pos error"(w1107) -> ()
                                n715 = Less?(x=w1107, y=3.0) -> (x < y?=w1109:bool)
                                n716 = Or(x=w1110, y=w1109) -> (x .or. y?=w1108:bool)
                                }
                                }
                                n717 = Index Array(array=w1084, index=3) -> (element=w1091:dbl)
                                n718 = global read "rio_Global.vi" "K"() -> (w1099:T27)
                                n719 = global read "rio_Global.vi" "H"() -> (w1098:T27)
                                n720 = global read "rio_Global.vi" "Pp"() -> (w1096:T27)
                                n721 = call-poly <vilib>:"Multiply.vi"("Real Matrix B"=w1098, "Real Matrix A"=w1099) -> ("A * B"=w1097:T27)
                                n722 = global read "rio_Global.vi" "Pp"() -> (w1094:T27)
                                n723 = call-poly <vilib>:"Multiply.vi"("Real Matrix B"=w1096, "Real Matrix A"=w1097) -> ("A * B"=w1095:T27)
                                n724 = call-poly <vilib>:"Subtract.vi"("Real Matrix B"=w1095, "Real Matrix A"=w1094) -> ("A - B"=w1093:T27)
                                n725 = global write "rio_Global.vi" "P"(w1093) -> ()
                                n726 = case shown="True" w1087 {
                                tunnel: w1091 -> [w1149 w1156]
                                tunnel: [w1149 w1151] -> w1085
                                frame False {
                                }
                                frame True {
                                n727 = global read "rio_Global.vi" "K"() -> (w1155:T27)
                                n728 = Index Array(array=w1155, index (row)=3, index (col)=2 ("disabled index (col)")) -> (element=w1152:dbl)
                                n729 = local read "h_gps"() -> (w1150:dbl)
                                n730 = call "headingweightsum2.vi"("a"=w1152, "h2"=w1150, "h1"=w1156) -> ("a*h2+(1-a)*h1"=w1151:dbl)  [unwired: 8 in]
                                }
                                }
                                n731 = case shown="True" w1086 {
                                tunnel: w1084 -> [w1125 w1137]
                                tunnel: [w1125 w1136] -> w1090
                                tunnel: w1085 -> [_ w1126]
                                frame False {
                                }
                                frame True {
                                n732 = disable-structure shown="Enabled" {
                                disable-tunnel: [w1147 w1148] -> w1127
                                disable-tunnel: w1126 -> [_ w1148]
                                frame Disabled {
                                n733 = local read "h_gps"() -> (w1147:dbl)
                                }
                                frame Enabled {
                                }
                                }
                                n734 = local read "pos_gps"() -> (w1131:dbl[])
                                n735 = call-poly <vilib>:"Array To Matrix.vi"("Real 1D Array"=w1137) -> ("Real Matrix (Column Vector)"=w1141:T27)
                                n736 = Array Subset(array=w1131, index=2, length=2) -> (w1132:dbl[])
                                n737 = Build Array (concatenate)(w1132, w1127) -> (w1128:dbl[])
                                n738 = global read "rio_Global.vi" "H"() -> (w1146:T27)
                                n739 = call-poly <vilib>:"Multiply.vi"("Real Matrix B"=w1141, "Real Matrix A"=w1146) -> ("A * B"=w1145:T27)
                                n740 = call-poly <vilib>:"Array To Matrix.vi"("Real 1D Array"=w1128) -> ("Real Matrix (Column Vector)"=w1144:T27)
                                n741 = call-poly <vilib>:"Subtract.vi"("Real Matrix B"=w1145, "Real Matrix A"=w1144) -> ("A - B"=w1142:T27)
                                n742 = global read "rio_Global.vi" "K"() -> (w1143:T27)
                                n743 = call-poly <vilib>:"Multiply.vi"("Real Matrix B"=w1142, "Real Matrix A"=w1143) -> ("A * B"=w1135:T27)
                                n744 = call-poly <vilib>:"Multiply.vi"("Real Matrix A"=w1135, "Real Scalar c"=0.25) -> ("c * A"=w1133:T27)
                                n745 = call-poly <vilib>:"Add.vi"("Real Matrix B"=w1141, "Real Matrix A"=w1133) -> ("A + B"=w1140:T27)
                                n746 = call-poly <vilib>:"Matrix To Array.vi"("Real Matrix"=w1140) -> ("Real 2D Array"=w1139:dbl[][])
                                n747 = Index Array(array=w1139, index (col)=0 ("disabled index (col)")) -> (element=w1136:dbl[])  [unwired: 1 in]
                                }
                                }
                                n748 = Replace Array Subset(array=w1090, new element=w1085, index=3) -> (w1088:dbl[])
                                }
                                }
                                }
                                }
                              }
                            }
                          }
                        }
                      }
                    }
                  }
                  frame #2 {
                    n749 = local read "h_gps"() -> (w1162:dbl)
                    n750 = local read "dt"() -> (w1159:dbl)
                    n751 = Index Array(array=w1173, index=3) -> (element=w1166:dbl)
                    n752 = Array Subset(array=w1173, index=0, length=2) -> (→"pos":dbl[])
                    n753 = Greater Than 0?(x=w1159) -> (x > 0?=w1158:bool)
                    n754 = call "angleconv.vi"("rad"=w1166) -> ("deg"=→"Heading":dbl)  [unwired: 9 in, 1 out]
                    n755 = Greater?(x=1.0, y=w1159) -> (0:w1161:bool)
                    n756 = call "headingoperater.vi"("h1"=0.0, "h2"=w1162) -> ("h2+h1"=w1163:dbl)  [unwired: 8 in, 1 out]
                    n757 = call "angleconv.vi"("rad"=w1163) -> ("deg"=→"H_GPS":dbl)  [unwired: 9 in, 1 out]
                    n758 = Compound Arithmetic op=AND(w1161, w1158) -> (w1157:bool)
                    n759 = case shown="True" w1157 {
                      tunnel: w1173 -> [_ w1174]
                      frame False {
                      }
                      frame True {
                        n760 = flat-sequence {
                          tunnel: w1174 -> [w1198]
                          frame #0 {
                            n761 = Get Date/Time In Seconds() -> (seconds since 1Jan1904=w1189:timestamp)
                            n762 = To Double Precision Float(number=w1189) -> (double precision float=w1183:dbl)
                            n763 = global read "rio_Global.vi" "LCM_POS_T"() -> (w1197:T28)
                            n764 = local read "POS init"() -> (w1179:bool)
                            n765 = Unbundle By Name(w1197) -> ("hash"=w1194:i64)
                            n766 = local read "dt"() -> (w1178:dbl)
                            n767 = Multiply(x=w1183, y=1000000.0) -> (x*y=w1181:dbl)
                            n768 = Array To Cluster(array=w1198) -> (cluster=w1196:T29)
                            n769 = Select(t=0.0, s=w1179, f=w1178) -> (s? t:f=w1176:dbl)
                            n770 = call "hash.vi"("input"=w1194) -> ("output"=w1193:i64)  [unwired: 10 in]
                            n771 = To Quad Integer(1:w1181) -> (0:w1180:i64)
                            n772 = Unbundle(w1196) -> ("Real 2D Array[0]"=w1188:dbl, "Real 2D Array[1]"=w1187:dbl, "Real 2D Array[2]"=w1186:dbl, "Real 2D Array[3]"=w1185:dbl, "Real 2D Array[4]"=w1184:dbl)
                            n773 = Bundle(cluster=w1197, "hash"=w1193, "sys time"=w1180, "dt"=w1176, "x"=w1188, "y"=w1187, "speed"=w1186, "heading"=w1185, "yaw_rate"=w1184) -> (w1175:T28)
                            n774 = Flatten To String(anything=w1175, prepend array or string size? (T)=FALSE) -> (data string=w1191:string)  [unwired: 2 in, 2 out]
                            n775 = global read "rio_Global.vi" "LCM"() -> (w1190:T5)
                            n776 = call "LCM_send.vi"("DATA"=w1191, "ID"="POS_T", "LCM"=w1190) -> ()  [unwired: 6 in, 3 out]
                          }
                        }
                      }
                    }
                  }
                }
              }
            }
            frame Disabled {
            }
          }
        }
      }
    }
    frame Disabled {
    }
  }
